vi "Process.vi"(8 "error in":errorcluster, 11 "LockinDAQ":refnum<class "LockinDAQ.lvclass">) -> (0 "error out":errorcluster, 3 "LockinDAQ out":refnum<class "LockinDAQ.lvclass">)   [LabVIEW 2016, in "LockinDAQ.lvclass"]
doc: "---------------------------------------------------------------\nJKI State Machine Objects™\nhttp://jki.net/state-machine-objects/\nCopyright (C) 2005-2015, JKI <info@jki.net>\nALL RIGHTS RESERVED"
uses:
  LockinDAQ.lvclass
  <vilib>/JKI/JKI SMO/SMO/SMO.lvclass
  <vilib>/JKI/JKI SMO/SMO/Typedefs/Parent Call--Enum.ctl
  Typedefs/State-enum.ctl
  Typedefs/Results--Cluster.ctl
  Typedefs/Sample Mode--Ring.ctl
  Typedefs/446xAO-enum.ctl
  Typedefs/DAQType-enum.ctl
  Typedefs/AO.config-cluster.ctl
  Typedefs/AO.config-array.ctl
  Typedefs/PrivateEvents--LockinDAQ.setAOconfig.ctl
  Typedefs/AI.coupling-enum.ctl
  Typedefs/446xAI-enum.ctl
  Typedefs/AI.config-cluster.ctl
  Typedefs/AI.config-array.ctl
  Typedefs/PrivateEvents--LockinDAQ.setAIconfig.ctl
  Typedefs/Function-enum.ctl
  Typedefs/AO-cluster.ctl
  Typedefs/PrivateEvents--LockinDAQ.setAO.ctl
  Typedefs/REF-cluster.ctl
  Typedefs/PrivateEvents--LockinDAQ.setREF.ctl
  Typedefs/Sampling.ctl
  Typedefs/PrivateEvents--LockinDAQ.setSampling.ctl
  Typedefs/Set State-enum.ctl
  Typedefs/PrivateEvents--LockinDAQ.setState.ctl
  Typedefs/PrivateEvents--LockinDAQ.setGain.ctl
  Typedefs/PrivateEvents--Cluster.ctl
  <vilib>/JKI/JKI SMO/SMO/Typedefs/StopProcessEventData--Cluster.ctl
  <vilib>/JKI/JKI SMO/SMO/Typedefs/AbortProcessEventData--Cluster.ctl
  <vilib>/JKI/JKI SMO/SMO/Typedefs/SMO Dependency Event--Enum.ctl
  <vilib>/JKI/JKI SMO/SMO/Typedefs/SMO Dependency Event--Cluster.ctl
  <vilib>/JKI/JKI SMO/SMO/Typedefs/Protected Events.ctl
  <resource>/objmgr/daqmx.rc
  Instrument.Lockin/Instrument.Lockin.lvclass
  Typedefs/PrivateEvents--LockinDAQ.setSweep.ctl
  Typedefs/Sweep Configuration--Cluster.ctl
  Typedefs/SweepResults--Cluster.ctl
  <userlib>/LevyLab/Levylab Instruments/SMOs/LevyLab/LevyLab.lvclass
  Typedefs/PrivateEvents--LockinDAQ.measureOffset.ctl
  Typedefs/PrivateEvents--LockinDAQ.zeroOffset.ctl
  <vilib>/measure/NI_MAPro.lvlib
  Typedefs/PrivateEvents--LockinDAQ.setPreFilter.ctl
  Typedefs/AI Prefilter-cluster.ctl
  C:/Program Files (x86)/National Instruments/LabVIEW 2016/vi.lib/JKI/JKI SMO/SMO/SMO.lvclass
  <vilib>/measure/madcrms.llb/Basic Averaged DC-RMS for N Chan.vi
panel:
  in  "Reset?":bool
  in  "zero offset":bool
  in  "measure offset":bool
  out "State":string
  out "Payload":variant
  out "DAQ Start Tasks (ms)":u32
  out "WFM Generation (ms)":u32
  out "Lockin (ms)":u32
  out "DAQ AO/AI (ms)":u32
  out "DAQ Create Tasks (ms)":u32
  in  "autophase?\n(experimental)":bool
  in  "reset REF":bool
  in  "60 Hz Prefilter?":bool
  in  "LP filter?":bool
  in  "LP Cutoff (Hz)":dbl=0.45 format="%#_13g"
  out "DAQ state":T1=enum."created"
  out "to":i32
  out "Method":string
  # "For instructions on how to use the JKI State Machine Objects, examples and video tutorials, visit:\nhttp://jki.net/state-machine-objects/\n\nJKI State Machine Objects™\nhttp://jki.net/state-machine-objects/\nCopyright (C) 2005-2015, JKI <info@jki.net>\nALL RIGHTS RESERVED"
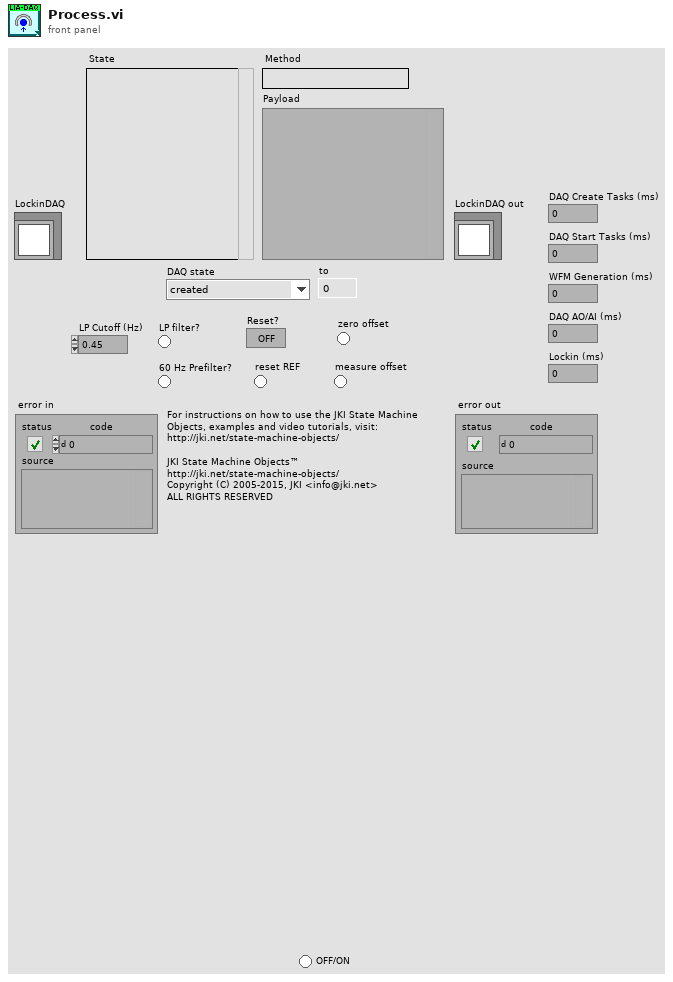
[diagram p1: front panel]
types:
  T1 = typedef "LockinDAQ.lvclass/State-enum.ctl" = enum16{"idle", "created", "started", "stopped", "sweeping"}
  T2 = typedef "SMO.lvclass/Parent Call--Enum.ctl" = enum16{"Allows parent to run", "Does not request parent to run"}
  T3 = enum32{"invalid app kind", "Development System", "Run Time System", "Student Edition", "Embedded LabVIEW", "Evaluation", "Custom"}
  T4 = enum32{"Invalid", "Standard", "Closed", "Hidden", "Minimized", "Maximized"}
  T5 = enum32{"Bad", "Idle", "Run top level", "Running"}
  T6 = typedef "LockinDAQ.lvclass/SweepResults--Cluster.ctl" = cluster{"Time Stamp":timestamp, "X Results":cluster{"parameter":dbl[], "x":dbl[]}[], "Y Results":cluster{"parameter":dbl[], "y":dbl[]}[]}
  T7 = typedef "LockinDAQ.lvclass/Sample Mode--Ring.ctl" = i32
  T8 = typedef "LockinDAQ.lvclass/AO.config-array.ctl" = T9[]
  T9 = typedef "LockinDAQ.lvclass/AO.config-cluster.ctl" = cluster{"AO.channels":tag, "AO.Range":T10, "output terminal configuration":i32, "DAQ Type":T11}
  T10 = typedef "LockinDAQ.lvclass/446xAO-enum.ctl" = enum16{"±0.1 V", "±1.0 V", "±10.0 V"}
  T11 = typedef "LockinDAQ.lvclass/DAQType-enum.ctl" = enum16{"None", "USB 4431", "PXI 446x"}
  T12 = typedef "LockinDAQ.lvclass/Results--Cluster.ctl" = cluster{"Time Stamp":timestamp, "Results":dbl[][]}
  T13 = cluster{"Core":cluster{"Current VI Reference":refnum<vi>, "Close Panel on Exit?":bool, "error":errorcluster}, "Self Reference":refnum<class "LockinDAQ.lvclass">, "to":i32, "state":T1, "sample mode":T7, "AO":waveform(dbl)[], "AI":waveform(dbl)[], "REF":waveform(dbl)[], "Results":T12, "sweep index":i32, "SweepResults [i]":T6, "SweepResults []":T6, "Offset":dbl[]}
  T14 = typedef "LockinDAQ.lvclass/AI.config-array.ctl" = T15[]
  T15 = typedef "LockinDAQ.lvclass/AI.config-cluster.ctl" = cluster{"AI.channels":tag, "AI.Coupling":T16, "AI.Range":T17, "input terminal configuration":i32, "DAQ Type":T11}
  T16 = typedef "LockinDAQ.lvclass/AI.coupling-enum.ctl" = u16
  T17 = typedef "LockinDAQ.lvclass/446xAI-enum.ctl" = enum16{"±0.316 V", "±1.00 V", "±3.16 V", "±10.0 V", "±31.6 V", "±42.4 V"}
  T18 = typedef "LockinDAQ.lvclass/AO-cluster.ctl" = cluster{"Ch":i32[], "Amp (V)":dbl[], "DC (V)":dbl[], "f (Hz)":dbl[], "Phase (°)":dbl[], "Function":T19[], "Sweep?":bool[]}
  T19 = typedef "LockinDAQ.lvclass/Function-enum.ctl" = enum16{"Sine", "Triangle", "Square", "Sawtooth"}
  T20 = typedef "LockinDAQ.lvclass/REF-cluster.ctl" = cluster{"Ch":i32[], " f (Hz)":dbl[], "Phase (°)":dbl[], "TC (s)":dbl[], "order":i32[]}
  T21 = typedef "LockinDAQ.lvclass/PrivateEvents--LockinDAQ.setGain.ctl" = dbl[]
  T22 = typedef "LockinDAQ.lvclass/Sampling.ctl" = cluster{"Fs":dbl, "#s":i32}
  T23 = cluster{"Sampling":T22, "Sample Mode":T7, "AI Buffer Size (S)":i32}
  T24 = typedef "LockinDAQ.lvclass/Sweep Configuration--Cluster.ctl" = cluster{"Sweep Time (s)":dbl, "Initial Wait Time (s)":dbl, "Sweep Channel":i32[], "Sweep Start (V)":dbl[], "Sweep End (V)":dbl[]}
  T25 = typedef "LockinDAQ.lvclass/AI Prefilter-cluster.ctl" = cluster{"60 Hz prefilter":bool, "LP prefilter":bool, "LP cutoff (Hz)":dbl}
  T26 = typedef "LockinDAQ.lvclass/Set State-enum.ctl" = enum16{"start", "stop", "reset", "calibrate", "start sweep", "stop sweep"}
  T27 = cluster{"Current VI Reference":refnum<vi>, "Close Panel on Exit?":bool, "error":errorcluster}
  T28 = typedef "SMO.lvclass/Protected Events.ctl" = cluster{"StopProcesses":refnum<user-event>, "AbortProcesses":refnum<user-event>, "Config Changed":refnum<user-event>, "Dependency":refnum<user-event>}
  T29 = typedef "LockinDAQ.lvclass/PrivateEvents--Cluster.ctl" = cluster{"setAOconfig":refnum<user-event>, "setAIconfig":refnum<user-event>, "setAO":refnum<user-event>, "setREF":refnum<user-event>, "setSampling":refnum<user-event>, "setState":refnum<user-event>, "setGain":refnum<user-event>, "setSweep":refnum<user-event>, "measureOffset":refnum<user-event>, "zeroOffset":refnum<user-event>, "setPreFilter":refnum<user-event>}
  T30 = cluster{"SMO":refnum<event-registration>, "LockinDAQ":refnum<event-registration>, "DAQmx":refnum<event-registration>}
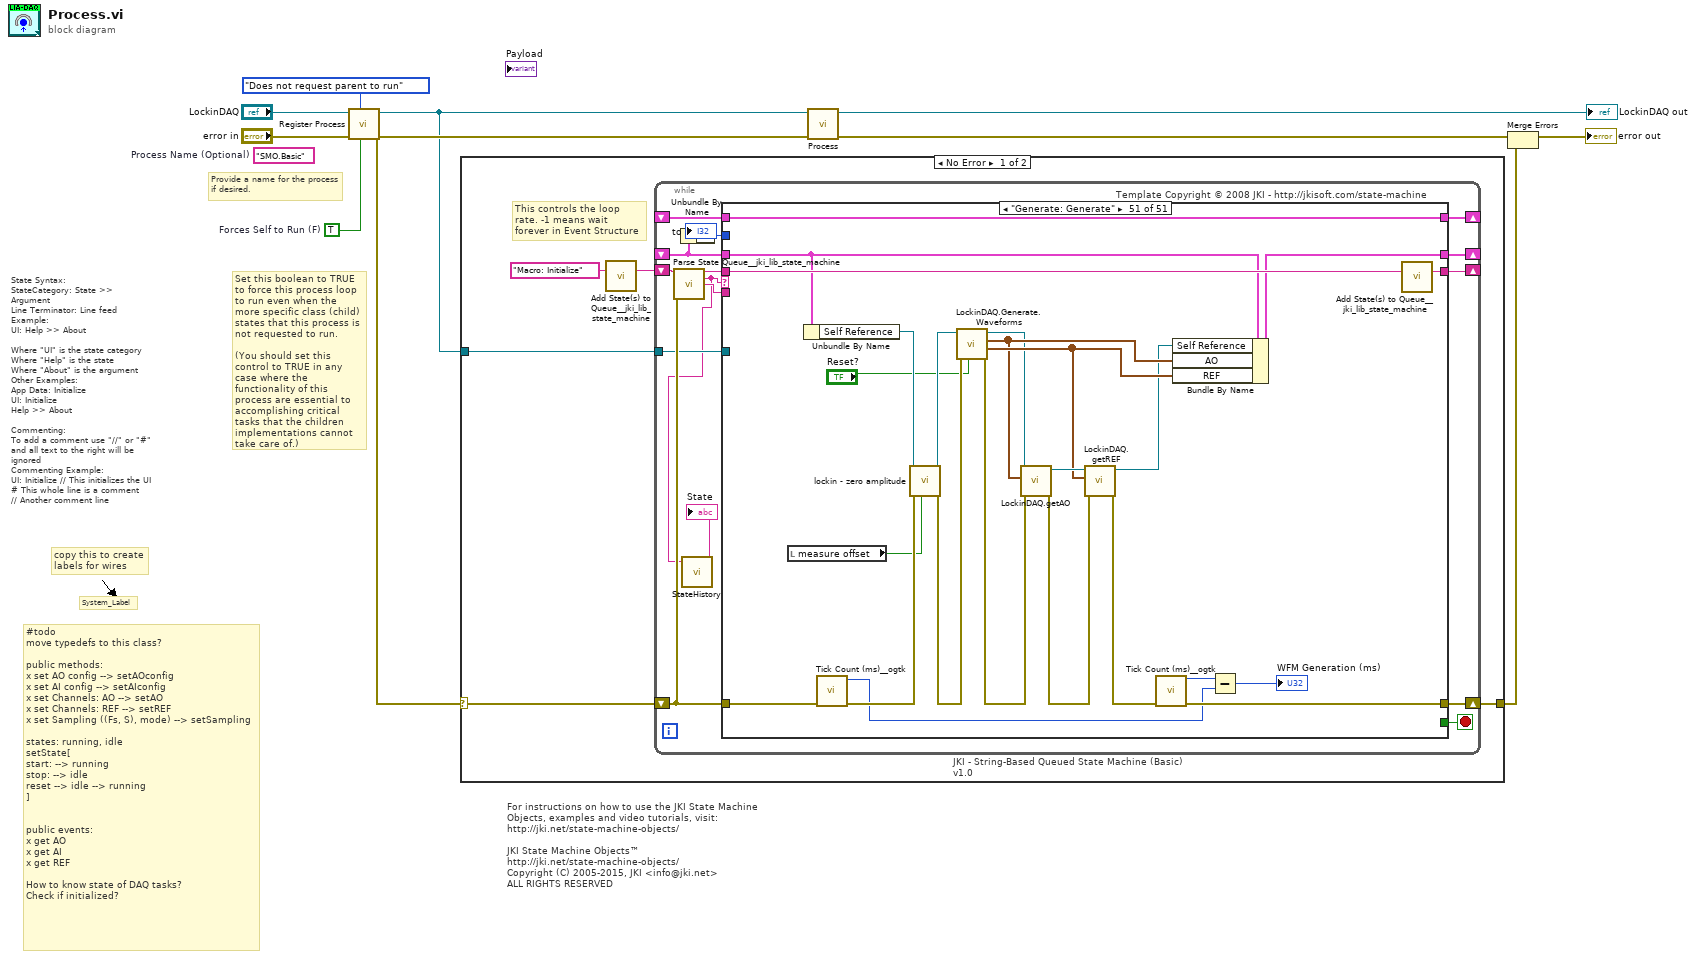
[diagram p0: block diagram]
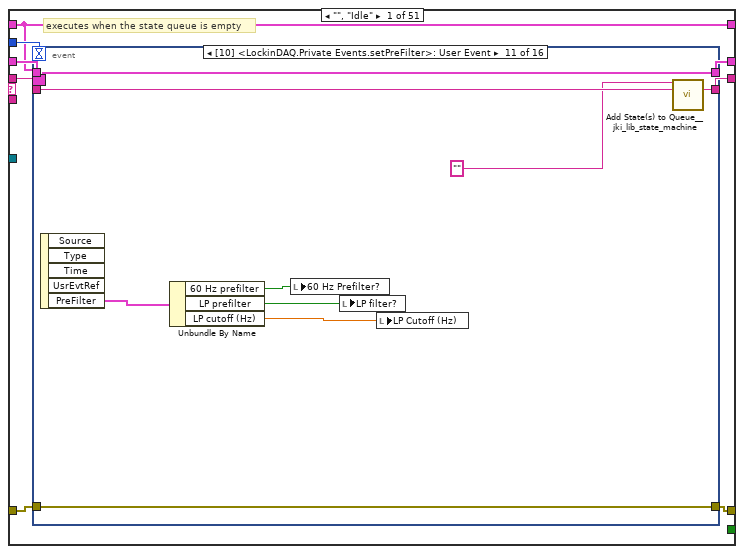
[diagram p2: hidden frame]
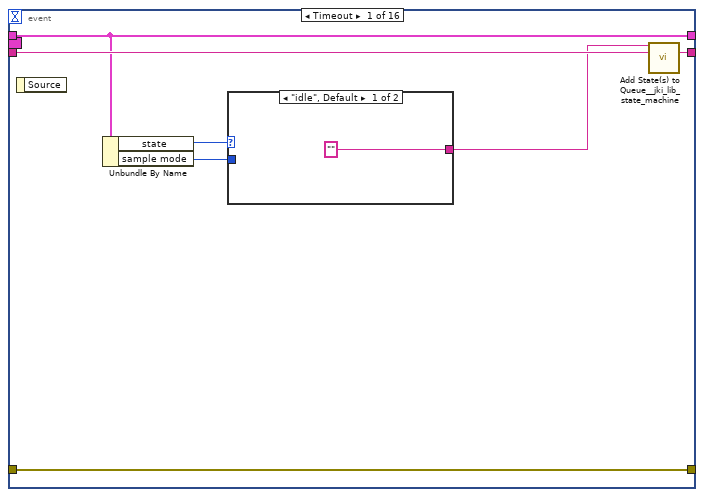
[diagram p3: hidden frame]
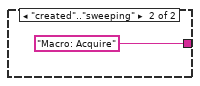
[diagram p4: hidden frame]
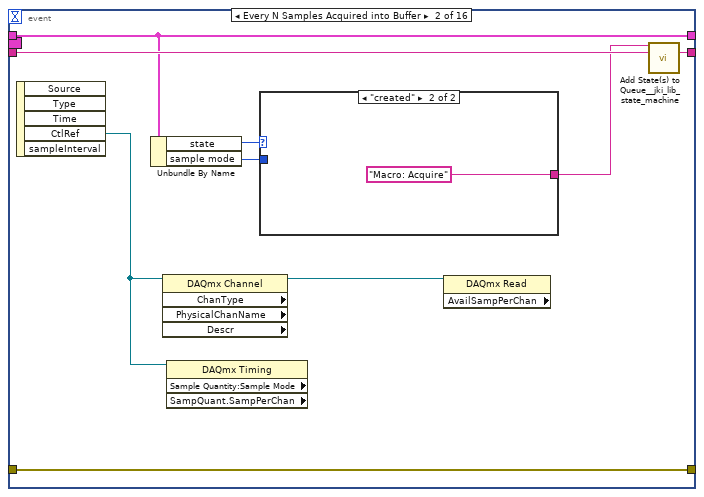
[diagram p5: hidden frame]
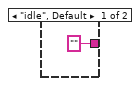
[diagram p6: hidden frame]
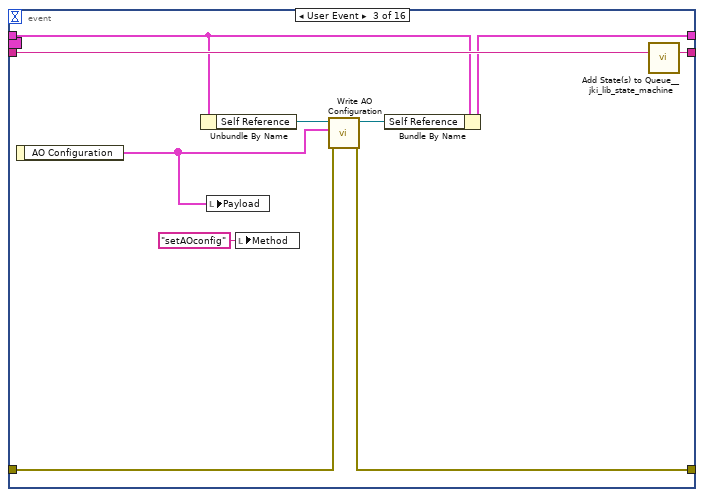
[diagram p7: hidden frame]
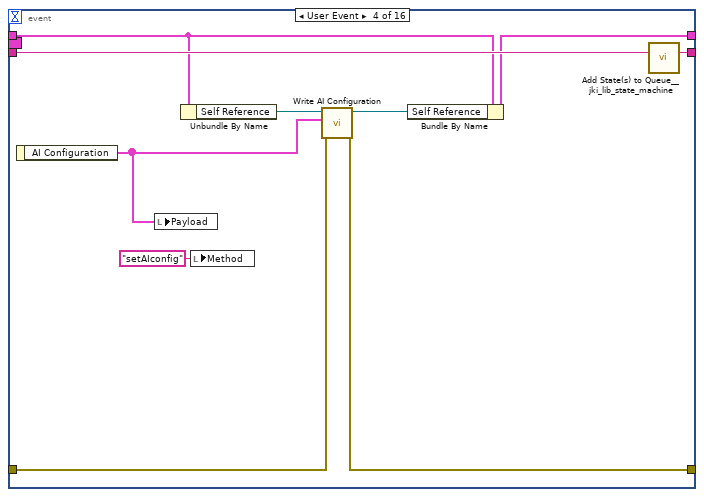
[diagram p8: hidden frame]
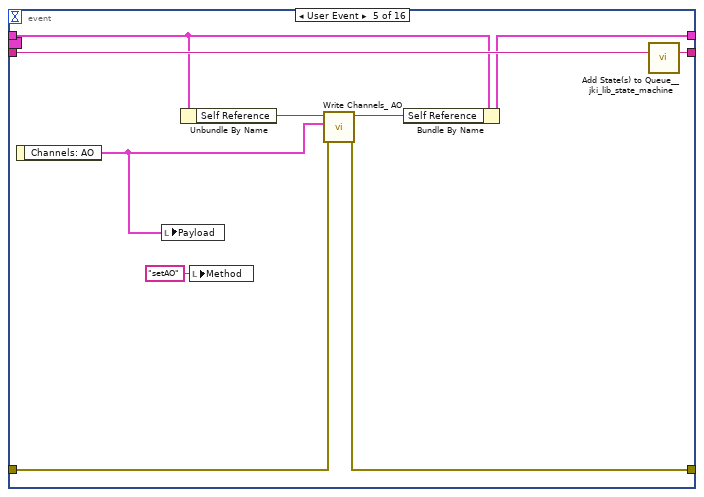
[diagram p9: hidden frame]
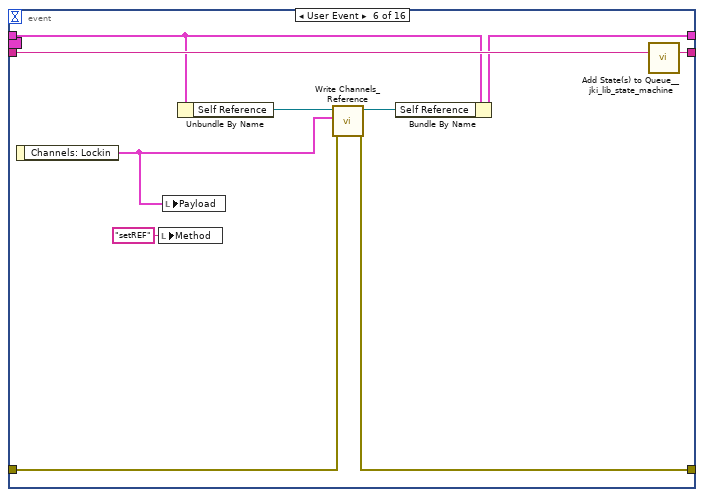
[diagram p10: hidden frame]
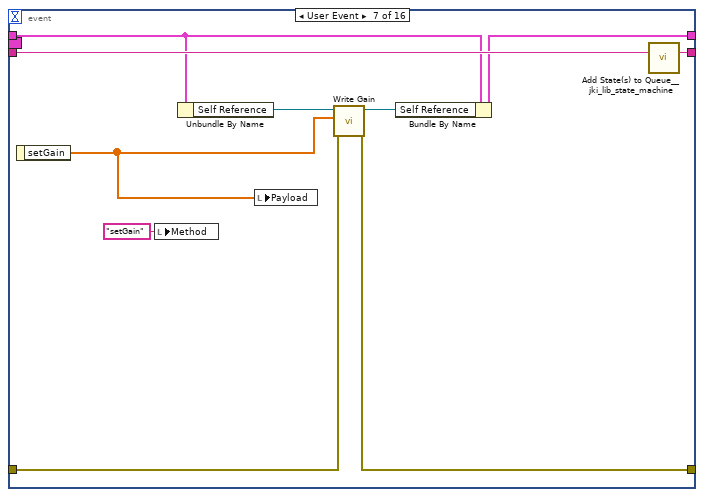
[diagram p11: hidden frame]
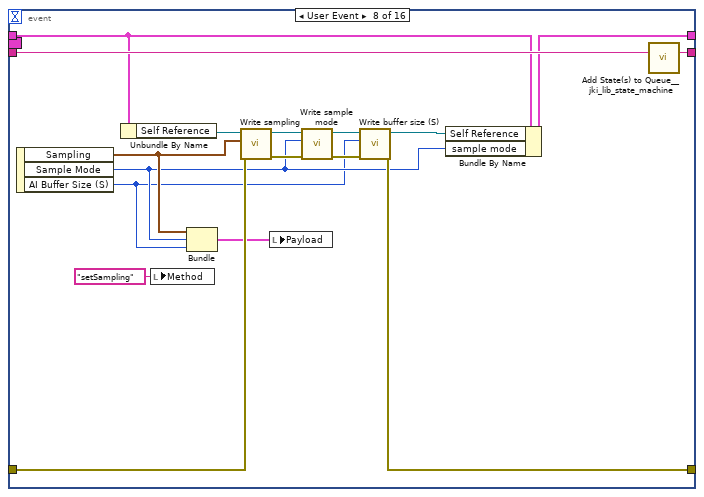
[diagram p12: hidden frame]
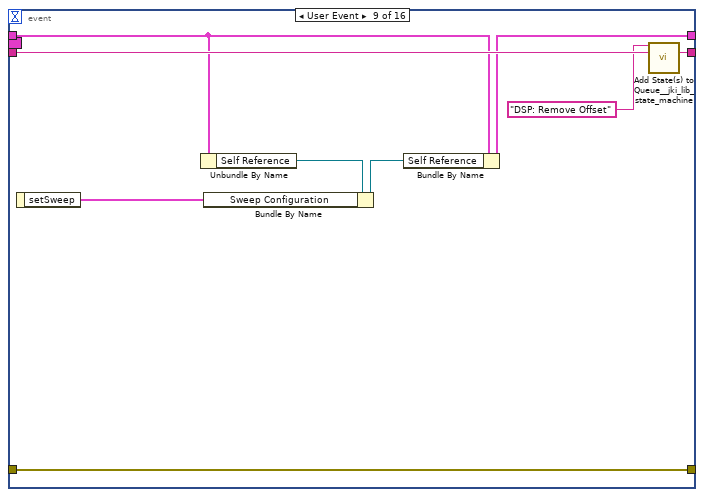
[diagram p13: hidden frame]
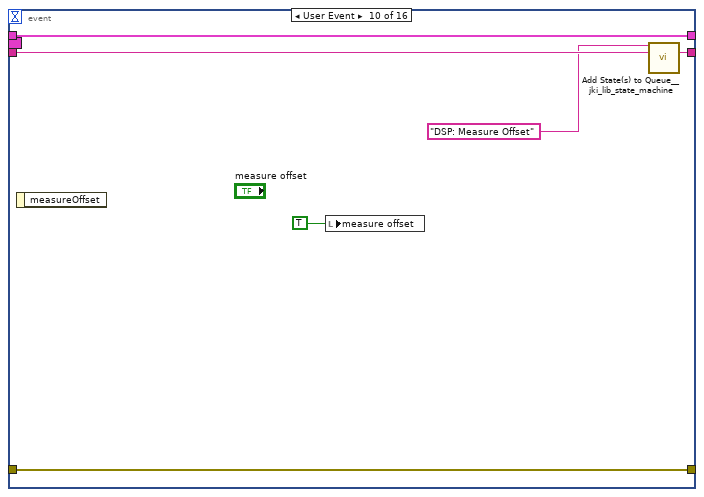
[diagram p14: hidden frame]
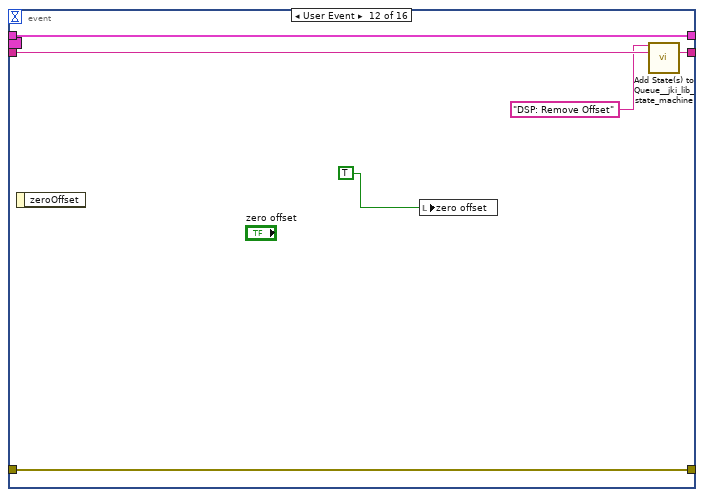
[diagram p15: hidden frame]
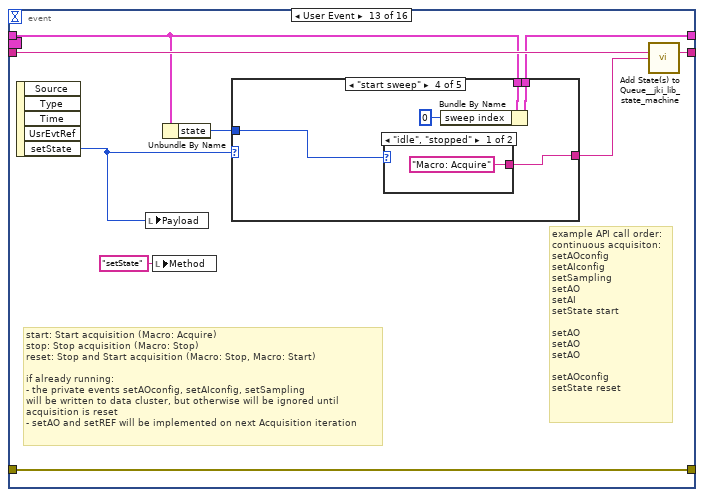
[diagram p16: hidden frame]
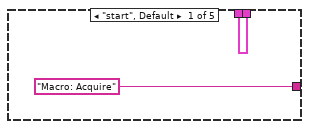
[diagram p17: hidden frame]
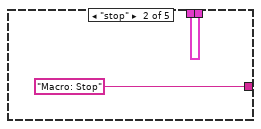
[diagram p18: hidden frame]
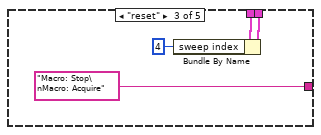
[diagram p19: hidden frame]
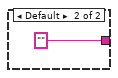
[diagram p20: hidden frame]
diagram:
  w1 = TRUE  # Forces Self to Run (F)
  (unwired) "SMO.Basic"  # Process Name (Optional)
  # "State Syntax:\nStateCategory: State >> Argument\nLine Terminator: Line feed\nExample:\nUI: Help >> About\n\nWhere \"UI\" is the state category\nWhere \"Help\" is the state\nWhere \"About\" is the argument\nOther Examples:\nApp Data: Initialize\nUI: Initialize\nHelp >> About\n\nCommenting:\nTo add a comment use \"//\" or \"#\" and all text to the right will be ignored\nCommenting Example:\nUI: Initialize // This initializes the UI\n# This whole line is a comment\n// Another comment line"
  # "copy this to create labels for wires"
  # "System_Label"
  # "#todo\nmove typedefs to this class?\n\npublic methods:\nx set AO config --> setAOconfig\nx set AI config --> setAIconfig\nx set Channels: AO --> setAO\nx set Channels: REF --> setREF\nx set Sampling ((Fs, S), mode) --> setSampling\n\nstates: running, idle\nsetState[\nstart: --> running\nstop: --> idle\nreset --> idle --> running\n]\n\n\npublic events:\nx get AO\nx get AI\nx get REF\n\nHow to know state of DAQ tasks?\nCheck if initialized?"
  # "Provide a name for the process\nif desired."
  # "Set this boolean to TRUE to force this process loop to run even when the more specific class (child) states that this process is not requested to run.\n\n(You should set this control to TRUE in any case where the functionality of this process are essential to accomplishing critical tasks that the children implementations cannot take care of.)"
  # "For instructions on how to use the JKI State Machine Objects, examples and video tutorials, visit:\nhttp://jki.net/state-machine-objects/\n\nJKI State Machine Objects™\nhttp://jki.net/state-machine-objects/\nCopyright (C) 2005-2015, JKI <info@jki.net>\nALL RIGHTS RESERVED"
  n1 = call <vilib>:"Register Process.vi"("Forces Self to Run (F)"=w1, "Parent Call"=Parent_Call--Enum."Does not request parent to run", "error in (no error)"="error in", "SMO"="LockinDAQ") -> ("error out"=w7:errorcluster, "SMO out"=w6:refnum<class "LockinDAQ.lvclass">)  [unwired: 6 in]
  n2 = case shown="No Error" w7 {
    selector: w7 -> [w14 w939]
    tunnel: w6 -> [w15 _]
    tunnel: [w13 w939] -> w3
    frame No Error {
      # "This controls the loop rate. -1 means wait forever in Event Structure"
      n3 = call <vilib>:"Add State(s) to Queue__jki_lib_state_machine.vi"("State(s) in (\"\")"="Macro: Initialize") -> ("States Out"=w12:string)  [unwired: 14 in]
      n4 = while "JKI - String-Based Queued State Machine (Basic) v1.0" {
        shift-right: [w25] -> _
        shift-left: _ -> [w19]
        shift-right: [w18] -> w13
        shift-left: w14 -> [w24]
        shift-right: [w27] -> _
        shift-left: w12 -> [w28]
        tunnel: w15 -> [w23]
        shift-right: [w22] -> _
        shift-left: _ -> [w21]
        stop <- w26 stop-if-true
        # "Template Copyright © 2008 JKI - http://jkisoft.com/state-machine"
        n5 = call <vilib>:"Parse State Queue__jki_lib_state_machine.vi"("State Queue"=w28, "Error In (no error)"=w24) -> ("Remaining States"=w30:string, "Current State"=w17:string, "Arguments"=w29:string)  [unwired: 11 in]
        n6 = Unbundle By Name(w19) -> ("to"=w20:i32)
        "to" <- w20
        n7 = call "StateHistory.vi"("Current State in"=w17) -> ("State History"=→"State":string)  [unwired: 8 in, 1 out]
        n8 = case shown="\"Generate: Generate\"" w17 {
          selector: w17 -> [_ _ w206 _ _ _ _ _ _ _ _ _ _ _ _ _ _ _ _ _ _ _ _ _ _ _ _ _ _ _ _ _ _ _ _ _ _ _ _ _ _ _ _ _ _ _ _ _ _ _ _]
          tunnel: w30 -> [w38 w204 w210 w229 w233 w254 w259 w281 w288 w293 w299 w306 w322 w354 w368 w382 w395 w405 w413 w421 w433 w438 w449 w454 w477 w483 w488 w505 w545 w583 w592 w602 w623 w660 w672 w677 w695 w738 w774 w789 w798 w804 w819 w828 w842 w854 w873 w892 w909 w914 w938]
          tunnel: w29 -> [_ _ _ _ _ _ _ _ _ _ _ w300 w316 _ _ _ _ _ _ _ _ _ _ _ _ _ _ _ _ _ _ w597 _ _ _ _ _ _ _ _ _ _ _ _ _ _ _ _ _ _ _]
          tunnel: w19 -> [w36 w201 w208 w220 w246 w250 w256 _ w283 w290 w297 w304 w318 w351 w364 w374 w390 w402 w406 w418 w431 w435 w446 w451 w475 w481 w486 w502 w542 w580 w590 w599 w620 w657 w663 w675 w682 w735 w771 w786 w792 w802 w816 w825 w831 w851 w859 w888 w905 w912 w934]
          tunnel: w24 -> [w34 w202 w211 w226 w239 _ w257 w279 w285 w291 w296 w302 w320 w352 w366 w380 w393 w403 w411 w414 w432 w436 w441 w452 w473 w480 w484 w499 w539 w578 w585 w594 w617 w654 w665 w673 w680 w723 w769 w777 w795 w800 w810 w823 w839 w848 w870 w883 w898 w910 w925]
          tunnel: [w37 w203 w209 w228 w230 w253 w258 w280 w287 w292 w298 w305 w321 w353 w367 w381 w394 w404 w412 w420 w429 w437 w448 w453 w476 w482 w487 w504 w544 w582 w591 w601 w622 w659 w671 w676 w694 w737 w773 w788 w797 w803 w818 w827 w841 w853 w872 w891 w908 w913 w937] -> w27
          tunnel: [_ _ _ _ _ TRUE _ _ _ _ _ _ _ _ _ _ _ _ _ _ _ _ _ _ _ _ _ _ _ _ _ _ _ _ _ _ _ _ _ _ _ _ _ _ _ _ _ _ _ _ _] -> w26
          tunnel: [w33 w201 w208 w227 w245 w250 w256 w270 w283 w290 w297 w304 w318 w351 w364 w374 w390 w402 w406 w418 w431 w435 w446 w451 w475 w481 w486 w501 w541 w579 w589 w598 w619 w656 w662 w675 w681 w734 w770 w785 w794 w802 w815 w824 w830 w850 w858 w889 w906 w912 w933] -> w25
          tunnel: w20 -> [w32 _ _ _ _ _ _ _ _ _ _ _ _ _ _ _ _ _ _ _ _ _ _ _ _ _ _ _ _ _ _ _ _ _ _ _ _ _ _ _ _ _ _ _ _ _ _ _ _ _ _]
          tunnel: w23 -> [_ _ _ _ _ _ _ w277 _ _ _ _ _ _ _ _ _ _ _ _ _ _ _ _ _ _ _ _ _ _ _ _ _ _ _ _ _ _ _ _ _ _ _ _ _ _ _ _ _ _ _]
          tunnel: [w31 w200 w205 w217 w248 w251 w255 w276 w282 w289 w295 w303 w315 w350 w365 w375 w392 w401 w410 w419 w430 w434 w447 w450 w468 w478 w485 w503 w543 w581 w588 w600 w621 w658 w669 w674 w693 w736 w772 w787 w796 w801 w817 w826 w840 w852 w871 w890 w907 w911 w936] -> w22
          tunnel: w21 -> [w31 w200 w205 w217 w248 w251 w255 w276 w282 w289 w295 w303 w315 w350 w365 w375 w392 w401 w410 w419 w430 w434 w447 w450 _ w478 w485 w503 w543 w581 w588 w600 w621 w658 w668 w674 w693 w736 w772 w787 w796 w801 w817 w826 w840 w852 w871 w890 w907 w911 w936]
          tunnel: [w35 w202 w212 w226 w247 w249 w257 w265 w284 w291 w296 w301 w319 w352 w366 w380 w393 w403 w411 w414 w432 w436 w440 w452 w472 w480 w484 w498 w538 w572 w584 w593 w612 w648 w664 w673 w679 w727 w763 w782 w795 w800 w814 w820 w839 w846 w870 w882 w904 w910 w920] -> w18
          frame "", "Idle" {
            # "executes when the state queue is empty"
            n9 = event shown="[10] <LockinDAQ.Private Events.setPreFilter>: User Event" {
              selector: w31 -> [_ _ _ _ _ _ _ _ _ _ _ _ _ _ _ _]
              dyn-events: _ -> [_ _ _ _ _ _ _ _ _ _ _ _ _ _ _ _]
              timeout: w32 -> [_ _ _ _ _ _ _ _ _ _ _ _ _ _ _ _]
              tunnel: w38 -> [w45 w56 w68 w78 w88 w98 w108 w125 w134 w140 w149 w155 w164 w189 w194 w199]
              tunnel: [w44 w55 w67 w77 w87 w97 w107 w124 w133 w139 w148 w154 w163 w188 w193 w198] -> w37
              tunnel: w36 -> [w42 w53 w64 w74 w84 w94 w104 w121 w130 w136 w145 w152 w157 w186 w191 w196]
              tunnel: [w43 w54 w60 w70 w80 w90 w101 w113 w131 w138 w147 w153 w162 w187 w192 w197] -> w35
              tunnel: w34 -> [w43 w54 w61 w71 w81 w91 w102 w117 w131 w138 w147 w153 w162 w187 w192 w197]
              tunnel: [w42 w53 w66 w76 w86 w96 w106 w123 w132 w136 w145 w152 w156 w186 w191 w196] -> w33
              event Timeout {
                n10 = event-data() -> ()  [unwired: 1 in, 1 out]
                n11 = Unbundle By Name(w42) -> ("state"=w40:T1, "sample mode"=w41:T7)
                n12 = case shown="\"idle\", Default" w40 {
                  tunnel: w41 -> [_ _]
                  tunnel: ["" ("State(s) in Front (\"\")") "Macro: Acquire" ("State(s) in Front (\"\")")] -> w39
                  frame "idle", Default {
                  }
                  frame "created".."sweeping" {
                  }
                }
                n13 = call <vilib>:"Add State(s) to Queue__jki_lib_state_machine.vi"("State(s) in Front (\"\")"=w39, "State(s) in (\"\")"=w45) -> ("States Out"=w44:string)  [unwired: 13 in]
              }
              event Every N Samples Acquired into Buffer {
                n14 = event-data() -> ("CtlRef"=w49:refnum<k21>)  [unwired: 1 in, 4 out]
                n15 = Unbundle By Name(w53) -> ("state"=w50:T1, "sample mode"=w52:T7)
                n16 = property class="DAQmx Channel" props=["ChanType", "PhysicalChanName", "Descr"](reference=w49) -> (reference out=w48:refnum<k21>)  [unwired: 1 in, 4 out]
                n17 = property class="DAQmx Timing" props=["Sample Quantity:Sample Mode", "SampQuant.SampPerChan"](reference=w49) -> ()  [unwired: 1 in, 4 out]
                n18 = case shown="\"created\"" w50 {
                  tunnel: w52 -> [_ _]
                  tunnel: ["" ("State(s) in Front (\"\")") "Macro: Acquire" ("State(s) in Front (\"\")")] -> w51
                  frame "idle", Default {
                  }
                  frame "created" {
                  }
                }
                n19 = property class="DAQmx Read" props=["AvailSampPerChan"](reference=w48) -> ()  [unwired: 1 in, 3 out]
                n20 = call <vilib>:"Add State(s) to Queue__jki_lib_state_machine.vi"("State(s) in Front (\"\")"=w51, "State(s) in (\"\")"=w56) -> ("States Out"=w55:string)  [unwired: 13 in]
              }
              event User Event {
                n21 = event-data() -> ("AO Configuration"=w59:T8)  [unwired: 1 in]
                n22 = Unbundle By Name(w64) -> ("Self Reference"=w63:refnum<class "LockinDAQ.lvclass">)
                n23 = local write "Payload"(w59) -> ()
                n24 = local write "Method"("setAOconfig" ("String")) -> ()
                n25 = call "Write AO Configuration.vi"("error in (no error)"=w61, "AO Configuration"=w59, "LockinDAQ"=w63) -> ("error out"=w60:errorcluster, "LockinDAQ out"=w62:refnum<class "LockinDAQ.lvclass">)  [unwired: 7 in]
                n26 = Bundle By Name(cluster=w64, "Self Reference"=w62) -> (w66:T13)
                n27 = call <vilib>:"Add State(s) to Queue__jki_lib_state_machine.vi"("State(s) in (\"\")"=w68) -> ("States Out"=w67:string)  [unwired: 14 in]
              }
              event User Event {
                n28 = event-data() -> ("AI Configuration"=w69:T14)  [unwired: 1 in]
                n29 = local write "Payload"(w69) -> ()
                n30 = Unbundle By Name(w74) -> ("Self Reference"=w73:refnum<class "LockinDAQ.lvclass">)
                n31 = local write "Method"("setAIconfig" ("String")) -> ()
                n32 = call "Write AI Configuration.vi"("error in (no error)"=w71, "AI Configuration"=w69, "LockinDAQ"=w73) -> ("error out"=w70:errorcluster, "LockinDAQ out"=w72:refnum<class "LockinDAQ.lvclass">)  [unwired: 7 in]
                n33 = Bundle By Name(cluster=w74, "Self Reference"=w72) -> (w76:T13)
                n34 = call <vilib>:"Add State(s) to Queue__jki_lib_state_machine.vi"("State(s) in (\"\")"=w78) -> ("States Out"=w77:string)  [unwired: 14 in]
              }
              event User Event {
                n35 = event-data() -> ("Channels: AO"=w79:T18)  [unwired: 1 in]
                n36 = local write "Payload"(w79) -> ()
                n37 = Unbundle By Name(w84) -> ("Self Reference"=w82:refnum<class "LockinDAQ.lvclass">)
                n38 = local write "Method"("setAO" ("String")) -> ()
                n39 = call "Write Channels_ AO.vi"("error in (no error)"=w81, "Channels: AO"=w79, "LockinDAQ"=w82) -> ("error out"=w80:errorcluster, "LockinDAQ out"=w83:refnum<class "LockinDAQ.lvclass">)  [unwired: 7 in]
                n40 = Bundle By Name(cluster=w84, "Self Reference"=w83) -> (w86:T13)
                n41 = call <vilib>:"Add State(s) to Queue__jki_lib_state_machine.vi"("State(s) in (\"\")"=w88) -> ("States Out"=w87:string)  [unwired: 14 in]
              }
              event User Event {
                n42 = event-data() -> ("Channels: Lockin"=w89:T20)  [unwired: 1 in]
                n43 = local write "Method"("setREF" ("String")) -> ()
                n44 = local write "Payload"(w89) -> ()
                n45 = Unbundle By Name(w94) -> ("Self Reference"=w93:refnum<class "LockinDAQ.lvclass">)
                n46 = call "Write Channels_ Reference.vi"("error in (no error)"=w91, "Channels: Lockin"=w89, "LockinDAQ"=w93) -> ("error out"=w90:errorcluster, "LockinDAQ out"=w92:refnum<class "LockinDAQ.lvclass">)  [unwired: 7 in]
                n47 = Bundle By Name(cluster=w94, "Self Reference"=w92) -> (w96:T13)
                n48 = call <vilib>:"Add State(s) to Queue__jki_lib_state_machine.vi"("State(s) in (\"\")"=w98) -> ("States Out"=w97:string)  [unwired: 14 in]
              }
              event User Event {
                n49 = event-data() -> ("setGain"=w99:T21)  [unwired: 1 in]
                n50 = local write "Method"("setGain" ("String")) -> ()
                n51 = Unbundle By Name(w104) -> ("Self Reference"=w103:refnum<class "LockinDAQ.lvclass">)
                n52 = local write "Payload"(w99) -> ()
                n53 = call "Write Gain.vi"("error in (no error)"=w102, "Gain"=w99, "LockinDAQ"=w103) -> ("error out"=w101:errorcluster, "LockinDAQ out"=w100:refnum<class "LockinDAQ.lvclass">)  [unwired: 7 in]
                n54 = Bundle By Name(cluster=w104, "Self Reference"=w100) -> (w106:T13)
                n55 = call <vilib>:"Add State(s) to Queue__jki_lib_state_machine.vi"("State(s) in (\"\")"=w108) -> ("States Out"=w107:string)  [unwired: 14 in]
              }
              event User Event {
                n56 = event-data() -> ("Sampling"=w112:T22, "Sample Mode"=w111:T7, "AI Buffer Size (S)"=w110:i32)  [unwired: 1 in]
                n57 = Unbundle By Name(w121) -> ("Self Reference"=w120:refnum<class "LockinDAQ.lvclass">)
                n58 = local write "Method"("setSampling" ("String")) -> ()
                n59 = Bundle("Sampling"=w112, "Sample Mode"=w111, "AI Buffer Size (S)"=w110) -> (w109:T23)  [unwired: 1 in]
                n60 = call "Write sampling.vi"("error in (no error)"=w117, "sampling"=w112, "LockinDAQ"=w120) -> ("error out"=w118:errorcluster, "LockinDAQ out"=w119:refnum<class "LockinDAQ.lvclass">)  [unwired: 7 in]
                n61 = local write "Payload"(w109) -> ()
                n62 = call "Write sample mode.vi"("error in (no error)"=w118, "sample mode"=w111, "LockinDAQ"=w119) -> ("error out"=w114:errorcluster, "LockinDAQ out"=w116:refnum<class "LockinDAQ.lvclass">)  [unwired: 7 in]
                n63 = call "Write buffer size (S).vi"("error in (no error)"=w114, "buffer size (S)"=w110, "LockinDAQ"=w116) -> ("error out"=w113:errorcluster, "LockinDAQ out"=w115:refnum<class "LockinDAQ.lvclass">)  [unwired: 7 in]
                n64 = Bundle By Name(cluster=w121, "Self Reference"=w115, "sample mode"=w111) -> (w123:T13)
                n65 = call <vilib>:"Add State(s) to Queue__jki_lib_state_machine.vi"("State(s) in (\"\")"=w125) -> ("States Out"=w124:string)  [unwired: 14 in]
              }
              event User Event {
                n66 = event-data() -> ("setSweep"=w127:T24)  [unwired: 1 in]
                n67 = Unbundle By Name(w130) -> ("Self Reference"=w129:refnum<class "LockinDAQ.lvclass">)
                n68 = Bundle By Name(cluster=w129, "Sweep Configuration"=w127) -> (w128:refnum<class "LockinDAQ.lvclass">)
                n69 = Bundle By Name(cluster=w130, "Self Reference"=w128) -> (w132:T13)
                n70 = call <vilib>:"Add State(s) to Queue__jki_lib_state_machine.vi"("State(s) in Front (\"\")"="DSP: Remove Offset" ("State(s) in Front (\"\")"), "State(s) in (\"\")"=w134) -> ("States Out"=w133:string)  [unwired: 13 in]
              }
              event User Event {
                n71 = event-data() -> ()  [unwired: 1 in, 1 out]
                n72 = local write "measure offset"(TRUE ("measureOffset")) -> ()
                n73 = call <vilib>:"Add State(s) to Queue__jki_lib_state_machine.vi"("State(s) in Front (\"\")"="DSP: Measure Offset" ("State(s) in Front (\"\")"), "State(s) in (\"\")"=w140) -> ("States Out"=w139:string)  [unwired: 13 in]
              }
              event User Event {
                n74 = event-data() -> ("PreFilter"=w144:T25)  [unwired: 1 in, 4 out]
                n75 = Unbundle By Name(w144) -> ("60 Hz prefilter"=w143:bool, "LP prefilter"=w142:bool, "LP cutoff (Hz)"=w141:dbl)
                n76 = local write "60 Hz Prefilter?"(w143) -> ()
                n77 = local write "LP filter?"(w142) -> ()
                n78 = local write "LP Cutoff (Hz)"(w141) -> ()
                n79 = call <vilib>:"Add State(s) to Queue__jki_lib_state_machine.vi"("State(s) in Front (\"\")"="" ("State(s) in Front (\"\")"), "State(s) in (\"\")"=w149) -> ("States Out"=w148:string)  [unwired: 13 in]
              }
              event User Event {
                n80 = event-data() -> ()  [unwired: 1 in, 1 out]
                n81 = local write "zero offset"(TRUE ("zero offset")) -> ()
                n82 = call <vilib>:"Add State(s) to Queue__jki_lib_state_machine.vi"("State(s) in Front (\"\")"="DSP: Remove Offset" ("State(s) in Front (\"\")"), "State(s) in (\"\")"=w155) -> ("States Out"=w154:string)  [unwired: 13 in]
              }
              event User Event {
                # "example API call order:\ncontinuous acquisiton:\nsetAOconfig\nsetAIconfig\nsetSampling\nsetAO\nsetAI\nsetState start\n\nsetAO\nsetAO\nsetAO\n\nsetAOconfig\nsetState reset"
                # "start: Start acquisition (Macro: Acquire)\nstop: Stop acquisition (Macro: Stop)\nreset: Stop and Start acquisition (Macro: Stop, Macro: Start)\n\nif already running:\n- the private events setAOconfig, setAIconfig, setSampling\nwill be written to data cluster, but otherwise will be ignored until\nacquisition is reset\n- setAO and setREF will be implemented on next Acquisition iteration"
                n83 = event-data() -> ("setState"=w158:T26)  [unwired: 1 in, 4 out]
                n84 = local write "Payload"(w158) -> ()
                n85 = local write "Method"("setState" ("String")) -> ()
                n86 = Unbundle By Name(w157) -> ("state"=w159:T1)
                n87 = case shown="\"start sweep\"" w158 {
                  tunnel: ["Macro: Acquire" ("State(s) in Front (\"\")") "Macro: Stop" ("State(s) in Front (\"\")") "Macro: Stop\nMacro: Acquire" ("State(s) in Front (\"\")") w175 "" ("State(s) in Front (\"\")")] -> w160
                  tunnel: w159 -> [_ _ _ w173 _]
                  tunnel: w157 -> [w165 w167 w172 w177 w183]
                  tunnel: [w165 w167 w171 w176 w182] -> w156
                  frame "start", Default {
                  }
                  frame "stop" {
                  }
                  frame "reset" {
                    n88 = Bundle By Name(cluster=w172, "sweep index"=4) -> (w171:T13)
                  }
                  frame "start sweep" {
                    n89 = case shown="\"idle\", \"stopped\"" w173 {
                      tunnel: ["Macro: Acquire" ("State(s) in Front (\"\")") "" ("State(s) in Front (\"\")")] -> w175
                      frame "idle", "stopped" {
                      }
                      frame Default {
                      }
                    }
                    n90 = Bundle By Name(cluster=w177, "sweep index"=0) -> (w176:T13)
                  }
                  frame "stop sweep" {
                    n91 = Bundle By Name(cluster=w183, "sweep index"=4) -> (w182:T13)
                  }
                }
                n92 = call <vilib>:"Add State(s) to Queue__jki_lib_state_machine.vi"("State(s) in (\"\")"=w164, "State(s) at Back (\"\")"=w160) -> ("States Out"=w163:string)  [unwired: 13 in]
              }
              event Panel Close? {
                # "Discard the event because we'll close the front panel ourselves in Macro: Exit"
                # "Close Panel button (pressed) Event\n(this executes Macro: Exit to terminate the VI)"
                n93 = event-data() -> ()  [unwired: 1 in, 1 out]
                n94 = event-data("Discard?"=FALSE) -> ()  [unwired: 1 in, 1 out]
                n95 = call <vilib>:"Add State(s) to Queue__jki_lib_state_machine.vi"("State(s) in Front (\"\")"="//Macro: Exit", "State(s) in (\"\")"=w189) -> ("States Out"=w188:string)  [unwired: 13 in]
              }
              event User Event {
                n96 = event-data() -> ()  [unwired: 1 in, 5 out]
                n97 = call <vilib>:"Add State(s) to Queue__jki_lib_state_machine.vi"("State(s) in Front (\"\")"="Macro: Exit", "State(s) in (\"\")"=w194) -> ("States Out"=w193:string)  [unwired: 13 in]
              }
              event User Event {
                # "On Abort, no nice macro exit, but exit right away"
                n98 = event-data() -> ()  [unwired: 1 in, 5 out]
                n99 = call <vilib>:"Add State(s) to Queue__jki_lib_state_machine.vi"("State(s) in Front (\"\")"="Exit", "State(s) in (\"\")"=w199) -> ("States Out"=w198:string)  [unwired: 13 in]
              }
            }
          }
          frame "---------- Core ----------" {
            # "Do not put any code in this frame.\n(it is a separator no-op)"
            n100 = call <vilib>:"Add State(s) to Queue__jki_lib_state_machine.vi"("State(s) in (\"\")"=w204) -> ("States Out"=w203:string)  [unwired: 14 in]
          }
          frame Default {
            w215 = 42 items=["No error", "Argument error", "Memory is full", "Out of zone", "End of file", "File already open", "Generic file I/O error", "File not found", "File permission error", "Disk is full", "Duplicate path", "Too many files open", "System feature not enabled", "Resource file not found", "Cannot add resource", "Resource not found", "Image not found", "Image memory error", "Pen does not exist", "Config type invalid", "Config token not found", "Config parse error", "Config memory error", "Bad external code format", "Bad external code offset", "External code not present", "Null window", "Destroy window error", "Null menu", "Print aborted", "Bad print record", "Print driver error", "Windows error during printing", "Memory error during printing", "Print dialog error", "Generic print error", "Invalid device refnum", "Device not found", "Device parameter error", "Device unit error", "Cannot open device", "Device call aborted", "Generic error", "Cancelled by user", "Object ID too low", "Object ID too high", "Object not in heap", "Unknown heap", "Unknown object (invalid DefProc)", "Unknown object (DefProc not in table)", "Message out of range", "Invalid (null) method", "Unknown message", "Manager call not supported", "Bad address", "Network operation in progress", "Network operation timed out", "Connection is busy", "Network attribute not supported", "Network error", "Address in use", "System out of memory", "Connection aborted", "Connection refused", "Not connected", "Already connected", "Connection closed", "Initialization error (interapplication manager)", "Bad occurrence", "Wait on unbound occurrence handler", "Occurrence queue overflow", "Datalog type conflict", "Unused", "Unrecognized type (interapplication manager)", "Memory corrupt", "Failed to make temporary DLL", "Old CIN version", "Drag socket not found", "Failed to load drop-object", "Failed to register OLE object", "Failed to release OLE object", "Format specifier type mismatch", "Unknown format specifier", "Too few format specifiers", "Too many format specifiers", "Scan failed", "Newer CIN version", "Error converting to variant", "Runtime menu error", "Password tampered", "Variant attribute not found", "Incompatible variant data type", "Event data is not available", "Event Store is not present", "Occurrence is not found", "Event Queue is not created", "Event info is not available", "Refnum passed is NULL", "Error retrieving Class GUID", "Error retrieving CoClass GUID", "Error retrieving TypeLib GUID.", "Bad built application magic bytes.", "Specific driver is different from the specific driver associated with the Logical Name.", "There is no session opened to the class driver.", "Max Error", "MAX - Error with config objects", "MAX - Error loading configuration", "MAX - Group not supported"]
            # "Current State"
            # "Do not delete, rename, or modify this frame.\n(this is used to capture unhandled states and typos)"
            # "Handle mistyped state name (developer tool)"
            n101 = Format Into String(format string="Software Exception: Unhandled State \"%s\"." ("message"), error in=w211, w206) -> (resulting string=w214:string, error out=w213:errorcluster)  [unwired: 1 in]
            n102 = call <vilib>:"Error Cluster From Error Code.vi"("show call chain? (False)"=TRUE, "error in (no error)"=w213, "error message (\"\")"=w214, "error code (0)"=w215) -> ("error out"=w212:errorcluster)  [unwired: 5 in]
            n103 = call <vilib>:"Add State(s) to Queue__jki_lib_state_machine.vi"("State(s) in (\"\")"=w210) -> ("States Out"=w209:string)  [unwired: 14 in]
          }
          frame "Initialize Core Data" {
            # "Do not delete, rename, or modify this frame.\n(this is used to determine panel behavior on exit)"
            # "originally closed?"
            # "exe?"
            # "If panel starts closed or is an EXE, then close it when we exit"
            n104 = property class="App"() -> ("App.Kind"=w224:T3)  [unwired: 2 in, 2 out]
            n105 = property class="VI"() -> ("Front Panel.Open"=w225:bool)  [unwired: 2 in, 2 out]
            n106 = control-ref of="Current VI Reference"() -> (w218:refnum<vi>)
            n107 = Not(x=w225) -> (.not. x?=w222:bool)
            n108 = Equal?(x=w224, y=T3."Run Time System" ("Application:Kind")) -> (x = y?=w221:bool)
            n109 = Or(x=w222, y=w221) -> (x .or. y?=w219:bool)
            n110 = Bundle By Name(cluster=w220, "Core.Current VI Reference"=w218, "Core.Close Panel on Exit?"=w219) -> (w227:T13)
            n111 = call <vilib>:"Add State(s) to Queue__jki_lib_state_machine.vi"("State(s) in (\"\")"=w229) -> ("States Out"=w228:string)  [unwired: 14 in]
          }
          frame "Error Handler" {
            w240 = FALSE  # Stop on Unhandled Error (T)
            w247 = errorcluster {"status"=FALSE, "code"=0, "source"=""}  # No error
            # "Overwrite this method to handle errors and pass to parent if not handled. Parent will fire a public event if the error is not handled up the chain of classes."
            n112 = Unbundle By Name(w246) -> ("Self Reference"=w237:refnum<class "LockinDAQ.lvclass">)
            n113 = call "LockinDAQ.ErrorHandler.vi"("error in (no error)"=w239, "LockinDAQ in"=w237) -> ("error out"=w238:errorcluster, "Error Filtered?"=w235:bool, "LockinDAQ out"=w236:refnum<class "LockinDAQ.lvclass">)  [unwired: 6 in, 1 out]
            n114 = call-dynamic "Handle Error.vi"("Stop on Unhandled Error (T)"=w240, "error in"=w238, "LevyLab"=w236) -> ("handling error"=w241:errorcluster, "Unhandled error"=w244:errorcluster)  [unwired: 6 in, 1 out]
            n115 = Bundle By Name(cluster=w246, "Core.error"=w244) -> (w245:T13)
            n116 = Select(t="Exit", s=w241, f="") -> (s? t:f=w232:string)
            n117 = call <vilib>:"Add State(s) to Queue__jki_lib_state_machine.vi"("State(s) in Front (\"\")"=w232, "State(s) in (\"\")"=w233) -> ("States Out"=w231:string)  [unwired: 13 in]
            n118 = Select(t="DAQ: STOP\nDAQ: CLEAR\nMacro: Acquire" ("States Out"), s=w235, f=w231) -> (s? t:f=w230:string)
          }
          frame "Exit" {
            # "Do not put any code in this frame.\n(No errors that occur here will be handled.)"
            n119 = Unbundle By Name(w250) -> ("Core.error"=w249:errorcluster)
            n120 = call <vilib>:"Add State(s) to Queue__jki_lib_state_machine.vi"("State(s) in (\"\")"=w254) -> ("States Out"=w253:string)  [unwired: 14 in]
          }
          frame "---------- Data ----------" {
            # "Do not put any code in this frame.\n(It is a separator no-op. You can make a copy of this frame to create a new Data frame)"
            n121 = call <vilib>:"Add State(s) to Queue__jki_lib_state_machine.vi"("State(s) in (\"\")"=w259) -> ("States Out"=w258:string)  [unwired: 14 in]
          }
          frame "Data: Initialize" {
            w260 = dbl[] []  # Offset
            w261 = T6 {"Time Stamp"=timestamp(0 s since 1904-01-01), "X Results"=[], "Y Results"=[]}  # SweepResults []
            w262 = T6 {"Time Stamp"=timestamp(0 s since 1904-01-01), "X Results"=[], "Y Results"=[]}  # SweepResults [i]
            w263 = -1  # sweep index
            w264 = T7 10178 items=["Finite Samples"=10178, "Continuous Samples"=10123]  # sample mode
            w269 = T12 {"Time Stamp"=timestamp(0 s since 1904-01-01), "Results"=[]}  # Results
            w268 = State-enum."idle"  # state
            w271 = -1  # to
            w272 = waveform(dbl)[] []  # REF
            w274 = waveform(dbl)[] []  # AO
            w273 = waveform(dbl)[] []  # AI
            w275 = T27 {"Current VI Reference"=refnum, "Close Panel on Exit?"=FALSE, "error"={"status"=FALSE, "code"=0, "source"=""}}  # Core
            w278 = refnum<class "LockinDAQ.lvclass"> refnum  # Self Reference
            # "start in idle mode"
            # "do not delete - used by framework"
            # "Data names and types of shift register data are defined by this bundle."
            # "Initialize the shift-register data, here.\n(data names are defined by what you wire into the bundle function)"
            n122 = Variant To Data(error in=w279, type=w278, Variant=w277) -> (data=w267:refnum<class "LockinDAQ.lvclass">, error out=w266:errorcluster)
            n123 = call "LockinDAQ.getDAQState.vi"("error in (no error)"=w266, "state"=w268, "LockinDAQ"=w267) -> ("error out"=w265:errorcluster)  [unwired: 7 in, 1 out]
            n124 = local write "DAQ state"(w268) -> ()
            n125 = Bundle("Core"=w275, "Self Reference"=w267, "to"=w271, "state"=w268, "sample mode"=w264, "AO"=w274, "AI"=w273, "REF"=w272, "Results"=w269, "sweep index"=w263, "SweepResults [i]"=w262, "SweepResults []"=w261, "Offset"=w260) -> (w270:T13)  [unwired: 1 in]
            n126 = call <vilib>:"Add State(s) to Queue__jki_lib_state_machine.vi"("State(s) in (\"\")"=w281) -> ("States Out"=w280:string)  [unwired: 14 in]
          }
          frame "Data: Cleanup" {
            # "Cleanup any data and references, here.\n(this is called automatically, by the Macro: Exit)"
            n127 = Unbundle By Name(w283) -> ("Core.Current VI Reference"=w286:refnum<vi>)
            n128 = Close Reference(reference=w286, error in (no error)=w285) -> (error out=w284:errorcluster)
            n129 = call <vilib>:"Add State(s) to Queue__jki_lib_state_machine.vi"("State(s) in (\"\")"=w288) -> ("States Out"=w287:string)  [unwired: 14 in]
          }
          frame "---------- UI ----------" {
            # "Do not put any code in this frame.\n(It is a separator no-op. You can make a copy of this frame to create a new UI frame)"
            n130 = call <vilib>:"Add State(s) to Queue__jki_lib_state_machine.vi"("State(s) in (\"\")"=w293) -> ("States Out"=w292:string)  [unwired: 14 in]
          }
          frame "UI: Initialize" {
            # "Initialize the User Interface, here.\n(this is called automatically, by the Macro: Init)"
            n131 = local write "Method"("" ("String")) -> ()
            n132 = call <vilib>:"Add State(s) to Queue__jki_lib_state_machine.vi"("State(s) in (\"\")"=w299) -> ("States Out"=w298:string)  [unwired: 14 in]
          }
          frame "UI: Cursor Set" {
            # "Argument"
            # "Initialize the User Interface, here.\n(this is called automatically, by the Macro: Init)"
            n133 = disable-structure shown="Default" {
              disable-tunnel: w302 -> [w307 w310]
              disable-tunnel: [w307 w309] -> w301
              disable-tunnel: w300 -> [_ w308]
              frame condition #0 {
              }
              frame condition #1 (active) {
                n134 = case shown="\"Idle\", Default" w308 {
                  tunnel: w310 -> [w312 w314]
                  tunnel: [w311 w313] -> w309
                  frame "Idle", Default {
                    n135 = call <vilib>:"Unset Busy.vi"("error in (no error)"=w312) -> ("error out"=w311:errorcluster)  [unwired: 10 in]
                  }
                  frame "Busy" {
                    n136 = call <vilib>:"Set Busy.vi"("error in (no error)"=w314) -> ("error out"=w313:errorcluster)  [unwired: 9 in, 1 out]
                  }
                }
              }
            }
            n137 = call <vilib>:"Add State(s) to Queue__jki_lib_state_machine.vi"("State(s) in (\"\")"=w306) -> ("States Out"=w305:string)  [unwired: 14 in]
          }
          frame "UI: Front Panel State" {
            # "Argument"
            # "Set Front Panel Open or Closed\n(Usage: \"UI: Front Panel State >> Open|Close\")"
            n138 = Unbundle By Name(w318) -> ("Core.Current VI Reference"=w317:refnum<vi>)
            n139 = disable-structure shown="Default" {
              disable-tunnel: w320 -> [w326 w349]
              disable-tunnel: [w325 w349] -> w319
              disable-tunnel: w317 -> [w324 _]
              disable-tunnel: w316 -> [w323 _]
              frame condition #0 (active) {
                n140 = case shown="\"Close\"" w323 {
                  tunnel: w326 -> [w330 w343]
                  tunnel: [w332 w344] -> w325
                  tunnel: w324 -> [w331 w341]
                  frame "Open", Default {
                    n141 = property class="VI"(reference=w331, error in=w330) -> (reference out=w328:refnum<vi>, error out=w329:errorcluster, "FP.State"=w327:T4)
                    n142 = case shown="\"Closed\"" w327 {
                      tunnel: [w335 w338] -> w332
                      tunnel: w329 -> [w334 w338]
                      tunnel: w328 -> [w333 _]
                      frame "Closed" {
                        n143 = invoke class="VI" method="FP.Open"(reference=w333, error in=w334, "Activate"=TRUE, "State"=T4."Standard") -> (error out=w335:errorcluster)  [unwired: 1 in, 4 out]
                      }
                      frame Default {
                      }
                    }
                  }
                  frame "Close" {
                    n144 = property class="VI"(reference=w341, error in=w343) -> (reference out=w340:refnum<vi>, error out=w342:errorcluster, "FP.State"=w339:T4)
                    n145 = case shown="Default" w339 {
                      tunnel: [w345 w348] -> w344
                      tunnel: w342 -> [w345 w347]
                      tunnel: w340 -> [_ w346]
                      frame "Invalid", "Closed" {
                      }
                      frame Default {
                        n146 = invoke class="VI" method="FP.Close"(reference=w346, error in=w347) -> (error out=w348:errorcluster)  [unwired: 1 in, 2 out]
                      }
                    }
                  }
                }
              }
              frame condition #1 {
              }
            }
            n147 = call <vilib>:"Add State(s) to Queue__jki_lib_state_machine.vi"("State(s) in (\"\")"=w322) -> ("States Out"=w321:string)  [unwired: 14 in]
          }
          frame "---------- Macro ----------" {
            # "Do not put any code in this frame.\n(It is a separator no-op. You can make a copy of this frame to create a new Macro frame)"
            n148 = call <vilib>:"Add State(s) to Queue__jki_lib_state_machine.vi"("State(s) in (\"\")"=w354) -> ("States Out"=w353:string)  [unwired: 14 in]
          }
          frame "Macro: Initialize" {
            w359 = "UI: Initialize\nUI: Front Panel State >> Open"  # UI: Initialize UI: Front Panel State >> Open
            w355 = "Process: Sync"
            # "Initialization Macro\n(This is called once, when the VI starts)"
            n149 = control-ref of="This VI"() -> (w357:refnum<vi>)
            n150 = property class="VI"(reference=w357) -> ("Exec.State"=w356:T5)  [unwired: 1 in, 2 out]
            n151 = Equal?(x=w356, y=T5."Run top level") -> (x = y?=w362:bool)
            n152 = Select(t=w355, s=w362, f="") -> ()  [unwired: 1 out]
            n153 = call <vilib>:"Add State(s) to Queue__jki_lib_state_machine.vi"("State(s) in Front (\"\")"="Data: Initialize\nInitialize Core Data\nEvents: Register", "State(s) in (\"\")"=w355, "State(s) at Back (\"\")"=w359) -> ("States Out"=w358:string)  [unwired: 12 in]
            n154 = call <vilib>:"Add State(s) to Queue__jki_lib_state_machine.vi"("State(s) in Front (\"\")"=w358, "State(s) in (\"\")"=w368) -> ("States Out"=w367:string)  [unwired: 13 in]
          }
          frame "Macro: Exit" {
            # "Exit Macro\n(This is called once, when the VI exits)"
            n155 = Unbundle By Name(w374) -> ("Core.Close Panel on Exit?"=w379:bool)
            n156 = Select(t="UI: Front Panel State >> Close", s=w379, f="") -> (s? t:f=w376:string)
            n157 = call <vilib>:"Add State(s) to Queue__jki_lib_state_machine.vi"("State(s) in Front (\"\")"="Macro: Stop\nData: Cleanup\nEvents: Unregister", "State(s) in (\"\")"="Process: Sync", "State(s) at Back (\"\")"="Exit") -> ("States Out"=w371:string)  [unwired: 12 in]
            n158 = call <vilib>:"Add State(s) to Queue__jki_lib_state_machine.vi"("State(s) in (\"\")"=w376, "State(s) at Back (\"\")"=w371) -> ("States Out"=w369:string)  [unwired: 13 in]
            n159 = call <vilib>:"Add State(s) to Queue__jki_lib_state_machine.vi"("State(s) in Front (\"\")"=w369, "State(s) in (\"\")"=w382) -> ("States Out"=w381:string)  [unwired: 13 in]
          }
          frame "Macro: Acquire" {
            (unwired) "DAQ: TIMED LOOP\nDAQ: STOP\nDAQ: CLEAR" ("State(s) in Front (\"\")")
            w391 = 10178 items=["Finite Samples"=10178, "Continuous Samples"=10123] ("sample mode")
            # "#todo:\ndo not create/clear tasks every time"
            # "note (8/23/2019):\nCREATE/START & STOP/CLEAR go hand-in-hand in the macro, but they are separated to make it easier to add features (e.g. event registration b/w CREATE and START)"
            # "already running = \nDAQmx tasks are STARTED"
            n160 = Unbundle By Name(w390) -> ("state"=w384:T1, "sample mode"=w387:T7)
            n161 = Equal?(x=w387, y=w391) -> (x = y?=w386:bool)
            n162 = case shown="\"idle\", Default" w384 {
              tunnel: ["DAQ: CREATE\n//DAQ: Event\nDAQ: START" ("State(s) in Front (\"\")") "" ("State(s) in Front (\"\")")] -> w388
              frame "idle", Default {
              }
              frame "created" {
              }
            }
            n163 = case shown="True" w386 {
              tunnel: ["" ("State(s) in Front (\"\")") "DAQ: STOP\nDAQ: CLEAR" ("State(s) in Front (\"\")")] -> w385
              frame False {
              }
              frame True {
              }
            }
            n164 = call <vilib>:"Add State(s) to Queue__jki_lib_state_machine.vi"("State(s) in Front (\"\")"=w388, "State(s) in (\"\")"="Macro: Generate\nDAQ: AO AI\nMacro: DSP\nMacro: Sweep" ("State(s) in Front (\"\")"), "State(s) at Back (\"\")"=w385) -> ("States Out"=w389:string)  [unwired: 12 in]
            n165 = call <vilib>:"Add State(s) to Queue__jki_lib_state_machine.vi"("State(s) in Front (\"\")"=w389, "State(s) in (\"\")"=w395) -> ("States Out"=w394:string)  [unwired: 13 in]
          }
          frame "Macro: Generate" {
            # "Do not put any code in this frame.\n(It is a separator no-op. You can make a copy of this frame to create a new Macro frame)"
            n166 = call <vilib>:"Add State(s) to Queue__jki_lib_state_machine.vi"("State(s) in Front (\"\")"="Generate: Generate" ("State(s) in Front (\"\")"), "State(s) in (\"\")"=w405) -> ("States Out"=w404:string)  [unwired: 13 in]
          }
          frame "Macro: DSP" {
            # "Do not put any code in this frame.\n(It is a separator no-op. You can make a copy of this frame to create a new Macro frame)"
            n167 = call <vilib>:"Add State(s) to Queue__jki_lib_state_machine.vi"("State(s) in Front (\"\")"="DSP: Phase" ("State(s) in Front (\"\")"), "State(s) at Back (\"\")"="DSP: Filter\nDSP: Lockin" ("State(s) in Front (\"\")")) -> ("States Out"=w408:string)  [unwired: 13 in]
            n168 = call <vilib>:"Add State(s) to Queue__jki_lib_state_machine.vi"("State(s) in Front (\"\")"=w408, "State(s) in (\"\")"=w413) -> ("States Out"=w412:string)  [unwired: 13 in]
          }
          frame "Macro: Sweep" {
            n169 = Unbundle By Name(w418) -> ("Self Reference"=w417:refnum<class "LockinDAQ.lvclass">, "sweep index"=w416:i32)
            n170 = case shown="4" w416 {
              tunnel: ["" ("State(s) in Front (\"\")") "Sweep: Initialize\nSweep: Set Initial\nSweep: Wait" ("State(s) in Front (\"\")") "Sweep: Wait" ("State(s) in Front (\"\")") "Sweep: Configure Sweep" ("State(s) in Front (\"\")") "Sweep: Save\nSweep: Done Sweeping?" ("State(s) in Front (\"\")") "Sweep: Stop" ("State(s) in Front (\"\")")] -> w415
              tunnel: w417 -> [_ _ _ _ _ _]
              frame -1, Default {
              }
              frame 0 {
              }
              frame 1 {
              }
              frame 2 {
              }
              frame 3 {
              }
              frame 4 {
              }
            }
            n171 = call <vilib>:"Add State(s) to Queue__jki_lib_state_machine.vi"("State(s) in Front (\"\")"=w415, "State(s) in (\"\")"=w421) -> ("States Out"=w420:string)  [unwired: 13 in]
          }
          frame "Macro: Stop" {
            n172 = call <vilib>:"Add State(s) to Queue__jki_lib_state_machine.vi"("State(s) in Front (\"\")"="DAQ: STOP\nDAQ: CLEAR" ("State(s) in Front (\"\")"), "State(s) in (\"\")"=w433) -> ("States Out"=w429:string)  [unwired: 13 in]
          }
          frame "---------- Process ----------" {
            # "Template Separator\n(You can make a copy of, or modify, this frame)"
            n173 = call <vilib>:"Add State(s) to Queue__jki_lib_state_machine.vi"("State(s) in (\"\")"=w438) -> ("States Out"=w437:string)  [unwired: 14 in]
          }
          frame "Process: Sync" {
            n174 = Unbundle By Name(w446) -> ("Self Reference"=w442:refnum<class "LockinDAQ.lvclass">)
            n175 = call <vilib>:"WaitOnProcessSync.vi"("error in (no error)"=w441, "SMO"=w442) -> ("error out"=w440:errorcluster, "Don't run?"=w445:bool)  [unwired: 7 in, 1 out]
            n176 = Select(t="Data: Cleanup\nEvents: Unregister\nExit", s=w445, f="") -> (s? t:f=w439:string)
            n177 = call <vilib>:"Add State(s) to Queue__jki_lib_state_machine.vi"("State(s) in Front (\"\")"=w439, "State(s) in (\"\")"=w449) -> ("States Out"=w448:string)  [unwired: 13 in]
          }
          frame "---------- Events ----------" {
            # "Template Separator\n(You can make a copy of, or modify, this frame)"
            n178 = call <vilib>:"Add State(s) to Queue__jki_lib_state_machine.vi"("State(s) in (\"\")"=w454) -> ("States Out"=w453:string)  [unwired: 14 in]
          }
          frame "Events: Register" {
            w455 = refnum<event-registration> refnum  # DAQmx
            w463 = refnum<event-registration> refnum  # SMO
            w464 = refnum<event-registration> refnum  # LockinDAQ
            # "Replace later"
            # "Expand to add\nmore events"
            n179 = Unbundle By Name(w475) -> ("Self Reference"=w474:refnum<class "LockinDAQ.lvclass">)
            n180 = call <vilib>:"GetProtectedEvents.vi"("SMO"=w474) -> ("error out"=w471:errorcluster, "SMO Protected Events"=w467:T28, "SMO out"=w470:refnum<class "LockinDAQ.lvclass">)  [unwired: 8 in]
            n181 = call "LockinDAQ.GetPrivateEvents.vi"("LockinDAQ"=w470) -> ("error out"=w457:errorcluster, "Private Events"=w466:T29)  [unwired: 8 in, 1 out]
            n182 = register-events(w467) -> (reference out=w469:refnum<event-registration>, error out=w462:errorcluster)  [unwired: 2 in]
            n183 = register-events(w466) -> (reference out=w465:refnum<event-registration>, error out=w459:errorcluster)  [unwired: 2 in]
            n184 = Variant To Data(error in=w459, type=w464, Variant=w465) -> (data=w456:refnum<event-registration>, error out=w460:errorcluster)
            n185 = Variant To Data(error in=w462, type=w463, Variant=w469) -> (data=w458:refnum<event-registration>, error out=w461:errorcluster)
            n186 = Bundle("SMO"=w458, "LockinDAQ"=w456, "DAQmx"=w455) -> (w468:T30)  [unwired: 1 in]
            n187 = Merge Errors(w461, w460, w457, w473, w471) -> (w472:errorcluster)
            n188 = call <vilib>:"Add State(s) to Queue__jki_lib_state_machine.vi"("State(s) in (\"\")"=w477) -> ("States Out"=w476:string)  [unwired: 14 in]
          }
          frame "Events: Unregister" {
            n189 = Unregister For Events(event registration refnum=w478, error in=w480) -> (error out=w479:errorcluster)
            n190 = call <vilib>:"Clear Errors.vi"("error in (no error)"=w479) -> ()  [unwired: 5 in, 2 out]
            n191 = call <vilib>:"Add State(s) to Queue__jki_lib_state_machine.vi"("State(s) in (\"\")"=w483) -> ("States Out"=w482:string)  [unwired: 14 in]
          }
          frame "---------- DAQ ----------" {
            n192 = call <vilib>:"Add State(s) to Queue__jki_lib_state_machine.vi"("State(s) in (\"\")"=w488) -> ("States Out"=w487:string)  [unwired: 14 in]
          }
          frame "DAQ: CREATE" {
            n193 = Unbundle By Name(w502) -> ("Self Reference"=w500:refnum<class "LockinDAQ.lvclass">, "state"=w490:T1)
            n194 = call <userlib>:"Tick Count (ms)__ogtk.vi"("error in (no error)"=w499) -> ("error out"=w493:errorcluster, "millisecond timer value"=w496:u32)  [unwired: 9 in]
            n195 = case shown="\"idle\"" w490 {
              selector: w490 -> [w509 _]
              tunnel: w500 -> [w508 w519]
              tunnel: [w508 w512] -> w494
              tunnel: w493 -> [w507 w518]
              tunnel: [w507 w513] -> w492
              tunnel: [w509 w511] -> w491
              tunnel: ["" ("State(s) in Front (\"\")") w510] -> w489
              frame Default {
              }
              frame "idle" {
                # "create DAQ tasks"
                n196 = call "LockinDAQ.Create.vi"("error in"=w518, "LockinDAQ"=w519) -> ("error out"=w515:errorcluster, "LockinDAQ out"=w514:refnum<class "LockinDAQ.lvclass">)  [unwired: 8 in]
                n197 = case shown="No Error" w515 {
                  selector: w515 -> [w522 w526]
                  tunnel: [State-enum."created" ("state") State-enum."idle" ("state")] -> w511
                  tunnel: [w522 w526] -> w516
                  tunnel: w514 -> [w521 w525]
                  tunnel: [w521 w525] -> w517
                  tunnel: ["" ("State(s) in Front (\"\")") "DAQ: CLEAR" ("State(s) in Front (\"\")")] -> w510
                  frame No Error {
                  }
                  frame Error {
                  }
                }
                n198 = call "LockinDAQ.getDAQState.vi"("error in (no error)"=w516, "state"=w511, "LockinDAQ"=w517) -> ("error out"=w513:errorcluster, "LockinDAQ out"=w512:refnum<class "LockinDAQ.lvclass">)  [unwired: 7 in]
              }
            }
            n199 = Bundle By Name(cluster=w502, "Self Reference"=w494, "state"=w491) -> (w501:T13)
            n200 = local write "DAQ state"(w491) -> ()
            n201 = call <userlib>:"Tick Count (ms)__ogtk.vi"("error in (no error)"=w492) -> ("error out"=w498:errorcluster, "millisecond timer value"=w497:u32)  [unwired: 9 in]
            n202 = Subtract(x=w497, y=w496) -> (x-y=→"DAQ Create Tasks (ms)":u32)
            n203 = call <vilib>:"Add State(s) to Queue__jki_lib_state_machine.vi"("State(s) in Front (\"\")"=w489, "State(s) in (\"\")"=w505) -> ("States Out"=w504:string)  [unwired: 13 in]
          }
          frame "DAQ: START" {
            n204 = Unbundle By Name(w542) -> ("to"=w528:i32, "Self Reference"=w540:refnum<class "LockinDAQ.lvclass">, "state"=w529:T1)
            n205 = call <userlib>:"Tick Count (ms)__ogtk.vi"("error in (no error)"=w539) -> ("error out"=w534:errorcluster, "millisecond timer value"=w536:u32)  [unwired: 9 in]
            n206 = case shown="\"started\", \"sweeping\"" w529 {
              selector: w529 -> [_ w566]
              tunnel: w540 -> [w555 w565]
              tunnel: w534 -> [w551 w567]
              tunnel: [w550 w567] -> w533
              tunnel: [w548 w565] -> w532
              tunnel: [w547 w564] -> w531
              tunnel: [w546 w566] -> w530
              tunnel: w528 -> [_ w564]
              frame Default {
                n207 = call "LockinDAQ.Start.vi"("error in"=w551, "LockinDAQ"=w555) -> ("error out"=w554:errorcluster, "LockinDAQ out"=w552:refnum<class "LockinDAQ.lvclass">)  [unwired: 8 in]
                n208 = case shown="No Error" w554 {
                  selector: w554 -> [w557 w561]
                  tunnel: [State-enum."started" ("state") State-enum."idle" ("state")] -> w546
                  tunnel: [1 -1] -> w547
                  tunnel: [w557 w561] -> w553
                  tunnel: w552 -> [w556 w560]
                  tunnel: [w556 w560] -> w549
                  frame No Error {
                  }
                  frame Error {
                  }
                }
                n209 = call "LockinDAQ.getDAQState.vi"("error in (no error)"=w553, "state"=w546, "LockinDAQ"=w549) -> ("error out"=w550:errorcluster, "LockinDAQ out"=w548:refnum<class "LockinDAQ.lvclass">)  [unwired: 7 in]
              }
              frame "started", "sweeping" {
              }
            }
            "DAQ state" <- w530
            n210 = Bundle By Name(cluster=w542, "to"=w531, "Self Reference"=w532, "state"=w530) -> (w541:T13)
            n211 = call <userlib>:"Tick Count (ms)__ogtk.vi"("error in (no error)"=w533) -> ("error out"=w538:errorcluster, "millisecond timer value"=w537:u32)  [unwired: 9 in]
            n212 = Subtract(x=w537, y=w536) -> (x-y=→"DAQ Start Tasks (ms)":u32)
            n213 = call <vilib>:"Add State(s) to Queue__jki_lib_state_machine.vi"("State(s) in (\"\")"=w545) -> ("States Out"=w544:string)  [unwired: 14 in]
          }
          frame "DAQ: AO AI" {
            # "write AO\nread AI"
            n214 = call <userlib>:"Tick Count (ms)__ogtk.vi"("error in (no error)"=w578) -> ("error out"=w573:errorcluster, "millisecond timer value"=w570:u32)  [unwired: 9 in]
            n215 = Unbundle By Name(w580) -> ("Self Reference"=w577:refnum<class "LockinDAQ.lvclass">, "AO"=w576:waveform(dbl)[])
            n216 = call "LockinDAQ.Read AI and Write AO.vi"("error in (no error)"=w573, "AO []"=w576, "LockinDAQ"=w577) -> ("error out"=w574:errorcluster, "AI []"=w568:waveform(dbl)[], "LockinDAQ out"=w575:refnum<class "LockinDAQ.lvclass">)  [unwired: 6 in]
            n217 = Bundle By Name(cluster=w580, "Self Reference"=w575, "AI"=w568) -> (w579:T13)
            n218 = call <userlib>:"Tick Count (ms)__ogtk.vi"("error in (no error)"=w574) -> ("error out"=w572:errorcluster, "millisecond timer value"=w571:u32)  [unwired: 9 in]
            n219 = Subtract(x=w571, y=w570) -> (x-y=→"DAQ AO/AI (ms)":u32)
            n220 = call <vilib>:"Add State(s) to Queue__jki_lib_state_machine.vi"("State(s) in (\"\")"=w583) -> ("States Out"=w582:string)  [unwired: 14 in]
          }
          frame "DAQ: TIMED LOOP" {
            # "!!!!!!!!!!!!!!!!!!!!!!!!!!!!!!!!!!!!!!!!!!!!!!!!!!!!!!!!!!!!!!!!!!!!!!!!\nTHIS IS AN EXPERIMENTAL BLOCKING CALL TO:\nGenerate\nRead/Write\nDSP\nIt should listen to events that change AO or REF Channels.\nInside there is a timed loop that will not stop unless it receives events for Set State = stop; SMO Stop; or SMO error\n!!!!!!!!!!!!!!!!!!!!!!!!!!!!!!!!!!!!!!!!!!!!!!!!!!!!!!!!!!!!!!!!!!!!!"
            n221 = Unbundle By Name(w590) -> ("Self Reference"=w587:refnum<class "LockinDAQ.lvclass">)
            n222 = call "LockinDAQ.TimedLoop.vi"("error in (no error)"=w585, "Event Cluster"=w588, "LockinDAQ"=w587) -> ("error out"=w584:errorcluster, "SMO out"=w586:refnum<class "LockinDAQ.lvclass">)  [unwired: 7 in]
            n223 = Bundle By Name(cluster=w590, "Self Reference"=w586) -> (w589:T13)
            n224 = call <vilib>:"Add State(s) to Queue__jki_lib_state_machine.vi"("State(s) in (\"\")"=w592) -> ("States Out"=w591:string)  [unwired: 14 in]
          }
          frame "DAQ: CALIBRATE" {
            # "calibrate or get calibration"
            n225 = Unbundle By Name(w599) -> ("Self Reference"=w596:refnum<class "LockinDAQ.lvclass">)
            n226 = case shown="\"False\", Default" w597 {
              tunnel: w596 -> [w606 w610]
              tunnel: [w605 w609] -> w595
              tunnel: w594 -> [w603 w608]
              tunnel: [w604 w607] -> w593
              frame "False", Default {
                n227 = call "LockinDAQ.Get Calibration.vi"("error in (no error)"=w603, "LockinDAQ"=w606) -> ("error out"=w604:errorcluster, "LockinDAQ out"=w605:refnum<class "LockinDAQ.lvclass">)  [unwired: 7 in, 1 out]
              }
              frame "True" {
                n228 = call "LockinDAQ.Calibrate.vi"("error in (no error)"=w608, "LockinDAQ"=w610) -> ("error out"=w607:errorcluster, "LockinDAQ out"=w609:refnum<class "LockinDAQ.lvclass">)  [unwired: 7 in, 1 out]
              }
            }
            n229 = Bundle By Name(cluster=w599, "Self Reference"=w595) -> (w598:T13)
            n230 = call <vilib>:"Add State(s) to Queue__jki_lib_state_machine.vi"("State(s) in (\"\")"=w602) -> ("States Out"=w601:string)  [unwired: 14 in]
          }
          frame "DAQ: STOP" {
            n231 = Unbundle By Name(w620) -> ("to"=w613:i32, "Self Reference"=w618:refnum<class "LockinDAQ.lvclass">, "state"=w616:T1)
            n232 = case shown="Default" w616 {
              selector: w616 -> [w625 w629]
              tunnel: w618 -> [w627 w637]
              tunnel: w617 -> [w624 w636]
              tunnel: [w627 w630] -> w615
              tunnel: [w626 w633] -> w614
              tunnel: w613 -> [w626 w628]
              tunnel: [w624 w632] -> w612
              tunnel: [w625 w631] -> w611
              frame "idle", "stopped" {
              }
              frame Default {
                # "stop DAQmx tasks"
                n233 = call "LockinDAQ.Stop.vi"("error in (no error)"=w636, "LockinDAQ"=w637) -> ("error out"=w635:errorcluster, "LockinDAQ out"=w634:refnum<class "LockinDAQ.lvclass">)  [unwired: 8 in]
                n234 = case shown="No Error" w635 {
                  selector: w635 -> [w641 w644]
                  tunnel: w634 -> [w642 w645]
                  tunnel: [-1 ("to") w646] -> w633
                  tunnel: [w640 w644] -> w632
                  tunnel: [w639 w647] -> w631
                  tunnel: [w638 w645] -> w630
                  tunnel: w629 -> [_ w647]
                  tunnel: w628 -> [_ w646]
                  frame No Error {
                    w639 = State-enum."stopped" ("state")
                    n235 = call "LockinDAQ.getDAQState.vi"("error in (no error)"=w641, "state"=w639, "LockinDAQ"=w642) -> ("error out"=w640:errorcluster, "LockinDAQ out"=w638:refnum<class "LockinDAQ.lvclass">)  [unwired: 7 in]
                  }
                  frame Error {
                  }
                }
              }
            }
            n236 = Bundle By Name(cluster=w620, "to"=w614, "Self Reference"=w615, "state"=w611) -> (w619:T13)
            n237 = local write "DAQ state"(w611) -> ()
            n238 = call <vilib>:"Add State(s) to Queue__jki_lib_state_machine.vi"("State(s) in (\"\")"=w623) -> ("States Out"=w622:string)  [unwired: 14 in]
          }
          frame "DAQ: CLEAR" {
            w649 = State-enum."idle" ("state")
            # "clear DAQmx tasks"
            n239 = Unbundle By Name(w657) -> ("Self Reference"=w655:refnum<class "LockinDAQ.lvclass">)
            n240 = call "LockinDAQ.Clear.vi"("error in (no error)"=w654, "LockinDAQ"=w655) -> ("error out"=w653:errorcluster, "LockinDAQ out"=w652:refnum<class "LockinDAQ.lvclass">)  [unwired: 8 in]
            n241 = call "LockinDAQ.getDAQState.vi"("error in (no error)"=w653, "state"=w649, "LockinDAQ"=w652) -> ("error out"=w648:errorcluster, "LockinDAQ out"=w650:refnum<class "LockinDAQ.lvclass">)  [unwired: 7 in]
            n242 = Bundle By Name(cluster=w657, "to"=-1, "Self Reference"=w650, "state"=w649) -> (w656:T13)
            n243 = local write "DAQ state"(w649) -> ()
            n244 = call <vilib>:"Add State(s) to Queue__jki_lib_state_machine.vi"("State(s) in (\"\")"=w660) -> ("States Out"=w659:string)  [unwired: 14 in]
          }
          frame "DAQ: Event" {
            # "Experimental state: generates a user event\nwhen there are a sufficient number of samples.\nUse to drive sequence instead of timeout"
            n245 = Unbundle By Name(w668) -> ("DAQmx"=w667:refnum<event-registration>)
            n246 = Unbundle By Name(w663) -> ("Self Reference"=w670:refnum<class "LockinDAQ.lvclass">)
            n247 = call "LockinDAQ.EventRegistration.vi"("error in (no error)"=w665, "DAQmx in"=w667, "LockinDAQ in"=w670) -> ("error out"=w664:errorcluster, "DAQmx out"=w666:refnum<event-registration>, "LockinDAQ out"=w661:refnum<class "LockinDAQ.lvclass">)  [unwired: 6 in]
            n248 = Bundle By Name(cluster=w663, "Self Reference"=w661) -> (w662:T13)
            n249 = Bundle By Name(cluster=w668, "DAQmx"=w666) -> (w669:T30)
            n250 = call <vilib>:"Add State(s) to Queue__jki_lib_state_machine.vi"("State(s) in (\"\")"=w672) -> ("States Out"=w671:string)  [unwired: 14 in]
          }
          frame "---------- DSP ----------" {
            n251 = call <vilib>:"Add State(s) to Queue__jki_lib_state_machine.vi"("State(s) in (\"\")"=w677) -> ("States Out"=w676:string)  [unwired: 14 in]
          }
          frame "DSP: Phase" {
            # "PRIVATE"
            # "PRIVATE"
            # "PRIVATE"
            # "PRIVATE"
            # "PRIVATE"
            n252 = Unbundle By Name(w682) -> ("Results"=w684:T12, "Self Reference"=w683:refnum<class "LockinDAQ.lvclass">)
            n253 = call "lockin - add phase element.vi"("error in (no error)"=w680, "LockinDAQ"=w683) -> ("error out"=w691:errorcluster, "LockinDAQ out"=w692:refnum<class "LockinDAQ.lvclass">)  [unwired: 8 in]
            n254 = case shown="True" "reset REF" {
              tunnel: w691 -> [w697 w701]
              tunnel: w692 -> [w696 w700]
              tunnel: [w697 w699] -> w689
              tunnel: [w696 w698] -> w688
              frame False {
              }
              frame True {
                n255 = call "lockin - Set REF phase equals zero.vi"("error in (no error)"=w701, "LockinDAQ out"=w700) -> ("error out"=w699:errorcluster, "LockinDAQ"=w698:refnum<class "LockinDAQ.lvclass">)  [unwired: 8 in]
              }
            }
            n256 = case shown="True" "autophase?\n(experimental)" {
              tunnel: w684 -> [_ w708]
              tunnel: w689 -> [w703 w707]
              tunnel: w688 -> [w702 w706]
              tunnel: [w703 w705] -> w687
              tunnel: [w702 w704] -> w685
              frame False {
              }
              frame True {
                n257 = call "4461 Autophase.vi"("error in (no error)"=w707, "Results"=w708, "LockinDAQ"=w706) -> ("error out"=w705:errorcluster, "LockinDAQ out"=w704:refnum<class "LockinDAQ.lvclass">)  [unwired: 7 in]
              }
            }
            n258 = call "4461 Replace AO Ch.vi"("error in (no error)"=w687, "LockinDAQ (NEW)"=w685, "LockinDAQ (OLD)"=w683) -> ("error out"=w679:errorcluster, "LockinDAQ out"=w678:refnum<class "LockinDAQ.lvclass">)  [unwired: 7 in]
            n259 = Bundle By Name(cluster=w682, "Self Reference"=w678) -> (w681:T13)
            n260 = call <vilib>:"Add State(s) to Queue__jki_lib_state_machine.vi"("State(s) in (\"\")"=w695) -> ("States Out"=w694:string)  [unwired: 14 in]
          }
          frame "DSP: Filter" {
            w717 = 1  # decimating factor
            w716 = FALSE  # averaging
            # "publish AI waveform"
            n261 = Unbundle By Name(w735) -> ("Self Reference"=w713:refnum<class "LockinDAQ.lvclass">, "AO"=w714:waveform(dbl)[], "REF"=w715:waveform(dbl)[], "AI"=w710:waveform(dbl)[], "Offset"=w709:dbl[])
            n262 = call "decimate_waveforms.vi"("decimating factor"=w717, "averaging"=w716, "error in (no error)"=w723, "WFM"=w714) -> ("error out"=w729:errorcluster, "WFM out"=w720:waveform(dbl)[])  [unwired: 6 in]
            n263 = call "decimate_waveforms.vi"("decimating factor"=w717, "averaging"=w716, "error in (no error)"=w723, "WFM"=w715) -> ("error out"=w730:errorcluster, "WFM out"=w721:waveform(dbl)[])  [unwired: 6 in]
            n264 = call "decimate_waveforms.vi"("decimating factor"=w717, "averaging"=w716, "error in (no error)"=w723, "WFM"=w710) -> ("error out"=w726:errorcluster, "WFM out"=w718:waveform(dbl)[])  [unwired: 6 in]
            n265 = Merge Errors(w729, w730, w726) -> (w712:errorcluster)
            n266 = call "Subtract Offset.vi"("error in (no error)"=w712, "Offset"=w709, "WFM in"=w718) -> ("error out"=w722:errorcluster, "WFM out"=w719:waveform(dbl)[])  [unwired: 7 in]
            n267 = case shown="True" "60 Hz Prefilter?" {
              tunnel: w719 -> [w747 w751]
              tunnel: [w747 w750] -> w732
              tunnel: w722 -> [w746 w749]
              tunnel: [w746 w748] -> w731
              frame False {
              }
              frame True {
                n268 = call "Prefilter_60Hz_Notch.vi"("error in (no error)"=w749, "Array in"=w751) -> ("error out"=w748:errorcluster, "Array out"=w750:waveform(dbl)[])  [unwired: 8 in]
              }
            }
            n269 = case shown="True" "LP filter?" {
              tunnel: w732 -> [w740 w745]
              tunnel: [w740 w741] -> w728
              tunnel: w731 -> [w739 w743]
              tunnel: [w739 w742] -> w711
              tunnel: "LP Cutoff (Hz)" -> [_ w744]
              frame False {
              }
              frame True {
                n270 = call "Prefilter_LP.vi"("error in (no error)"=w743, "high cutoff freq [Hz]"=w744, "WFM in"=w745) -> ("error out"=w742:errorcluster, "WFM out"=w741:waveform(dbl)[])  [unwired: 7 in]
              }
            }
            n271 = Bundle By Name(cluster=w735, "AO"=w720, "REF"=w721, "AI"=w728) -> (w734:T13)
            n272 = call "LockinDAQ.getAI.vi"("error in (no error)"=w711, "getAI"=w728, "LockinDAQ"=w713) -> ("error out"=w727:errorcluster)  [unwired: 7 in, 1 out]
            n273 = call <vilib>:"Add State(s) to Queue__jki_lib_state_machine.vi"("State(s) in (\"\")"=w738) -> ("States Out"=w737:string)  [unwired: 14 in]
          }
          frame "DSP: Lockin" {
            # "publish Results"
            # "lockin demodulation"
            n274 = Unbundle By Name(w771) -> ("Self Reference"=w754:refnum<class "LockinDAQ.lvclass">, "AI"=w756:waveform(dbl)[], "REF"=w752:waveform(dbl)[])
            n275 = call <userlib>:"Tick Count (ms)__ogtk.vi"("error in (no error)"=w769) -> ("error out"=w758:errorcluster, "millisecond timer value"=w761:u32)  [unwired: 9 in]
            n276 = call "Divide Gain.vi"("error in (no error)"=w758, "WFM in"=w756, "LockinDAQ"=w754) -> ("error out"=w757:errorcluster, "WFM out"=w759:waveform(dbl)[], "LockinDAQ out"=w753:refnum<class "LockinDAQ.lvclass">)  [unwired: 6 in]
            n277 = call "Lockin Engine.vi"("error in (no error)"=w757, "REF Waveforms"=w752, "AI Waveforms"=w759, "LockinDAQ"=w753) -> ("error out"=w765:errorcluster, "SweepResults"=w755:T6, "Averaged Results (X,Y,R,Theta,Mean)"=w766:T12, "LockinDAQ out"=w768:refnum<class "LockinDAQ.lvclass">)  [unwired: 4 in]
            n278 = call "LockinDAQ.getResults.vi"("error in (no error)"=w765, "Results"=w766, "LockinDAQ"=w768) -> ("error out"=w764:errorcluster, "LockinDAQ out"=w767:refnum<class "LockinDAQ.lvclass">)  [unwired: 7 in]
            n279 = Bundle By Name(cluster=w771, "Self Reference"=w767, "Results"=w766, "SweepResults [i]"=w755) -> (w770:T13)
            n280 = call <userlib>:"Tick Count (ms)__ogtk.vi"("error in (no error)"=w764) -> ("error out"=w763:errorcluster, "millisecond timer value"=w762:u32)  [unwired: 9 in]
            n281 = Subtract(x=w762, y=w761) -> (x-y=→"Lockin (ms)":u32)
            n282 = call <vilib>:"Add State(s) to Queue__jki_lib_state_machine.vi"("State(s) in (\"\")"=w774) -> ("States Out"=w773:string)  [unwired: 14 in]
          }
          frame "DSP: Measure Offset" {
            # "remove any existing offset\nbefore calculating new offset"
            # "reset indicator after measuring"
            n283 = Unbundle By Name(w786) -> ("AI"=w775:waveform(dbl)[], "Offset"=w780:dbl[])
            n284 = Negate(x=w780) -> (-x=w779:dbl[])
            n285 = call "Subtract Offset.vi"("error in (no error)"=w777, "Offset"=w779, "WFM in"=w775) -> ("error out"=w776:errorcluster, "WFM out"=w778:waveform(dbl)[])  [unwired: 7 in]
            n286 = call-poly <vilib>:"Basic Averaged DC-RMS.vi"("reset"=TRUE, "error in (no error)"=w776, "signals in"=w778) -> ("error out"=w782:errorcluster, "DC values"=w784:dbl[])  [unwired: 5 in, 2 out]
            n287 = Bundle By Name(cluster=w786, "Offset"=w784) -> (w785:T13)
            n288 = local write "measure offset"(FALSE ("measureOffset")) -> ()
            n289 = call <vilib>:"Add State(s) to Queue__jki_lib_state_machine.vi"("State(s) in (\"\")"=w789) -> ("States Out"=w788:string)  [unwired: 14 in]
          }
          frame "DSP: Remove Offset" {
            # "reset indicator after zeroing"
            n290 = Unbundle By Name(w792) -> ("AI"=w791:waveform(dbl)[])
            n291 = for {
              tunnel: w791 -> [_] mode=indexing
              tunnel: [0.0] -> w790 mode=indexing
            }
            n292 = local write "zero offset"(FALSE ("measureOffset")) -> ()
            n293 = Bundle By Name(cluster=w792, "Offset"=w790) -> (w794:T13)
            n294 = call <vilib>:"Add State(s) to Queue__jki_lib_state_machine.vi"("State(s) in (\"\")"=w798) -> ("States Out"=w797:string)  [unwired: 14 in]
          }
          frame "---------- Sweep ----------" {
            n295 = call <vilib>:"Add State(s) to Queue__jki_lib_state_machine.vi"("State(s) in (\"\")"=w804) -> ("States Out"=w803:string)  [unwired: 14 in]
          }
          frame "Sweep: Initialize" {
            w813 = State-enum."sweeping" ("state")
            n296 = Unbundle By Name(w816) -> ("Self Reference"=w809:refnum<class "LockinDAQ.lvclass">)
            n297 = Unbundle By Name(w809) -> ("Channels: AO"=w808:T18)
            n298 = Bundle By Name(cluster=w809, "Saved Channels: AO"=w808) -> (w811:refnum<class "LockinDAQ.lvclass">)
            n299 = Get Date/Time In Seconds() -> (seconds since 1Jan1904=w806:timestamp)
            n300 = Bundle By Name(cluster=T6 {"Time Stamp"=timestamp(0 s since 1904-01-01), "X Results"=[], "Y Results"=[]} ("All Results []"), "Time Stamp"=w806) -> (w805:T6)
            n301 = Bundle By Name(cluster=w816, "Self Reference"=w811, "SweepResults []"=w805, "state"=w813, "sweep index"=0) -> (w815:T13)
            n302 = call "LockinDAQ.getDAQState.vi"("error in (no error)"=w810, "state"=w813, "LockinDAQ"=w811) -> ("error out"=w814:errorcluster)  [unwired: 7 in, 1 out]
            n303 = call <vilib>:"Add State(s) to Queue__jki_lib_state_machine.vi"("State(s) in (\"\")"=w819) -> ("States Out"=w818:string)  [unwired: 14 in]
          }
          frame "Sweep: Set Initial" {
            # "1: Set Initial Vstart"
            n304 = Unbundle By Name(w825) -> ("Self Reference"=w821:refnum<class "LockinDAQ.lvclass">)
            n305 = call "LockinDAQ.Set Initial Value.vi"("error in (no error)"=w823, "LockinDAQ in"=w821) -> ("error out"=w820:errorcluster, "LockinDAQ out"=w822:refnum<class "LockinDAQ.lvclass">)  [unwired: 8 in]
            n306 = Bundle By Name(cluster=w825, "Self Reference"=w822) -> (w824:T13)
            n307 = call <vilib>:"Add State(s) to Queue__jki_lib_state_machine.vi"("State(s) in (\"\")"=w828) -> ("States Out"=w827:string)  [unwired: 14 in]
          }
          frame "Sweep: Wait" {
            n308 = Unbundle By Name(w831) -> ("sweep index"=w836:i32, "Self Reference"=w829:refnum<class "LockinDAQ.lvclass">)
            n309 = Unbundle By Name(w829) -> ("Initial Wait Time (s)"=w837:dbl)
            n310 = Equal To 0?(x=w836) -> (x = 0?=w835:bool)
            n311 = Multiply(x=w837, y=1000.0) -> (x*y=w833:dbl)
            n312 = call <userlib>:"Periodic Trigger__ogtk.vi"("time (ms)"=w833, "reset"=w835) -> ("Triggered"=w834:bool)  [unwired: 11 in, 2 out]
            n313 = case shown="True" w834 {
              tunnel: [1 ("sweep index") 2 ("sweep index")] -> w832
              frame False {
              }
              frame True {
              }
            }
            n314 = Bundle By Name(cluster=w831, "sweep index"=w832) -> (w830:T13)
            n315 = call <vilib>:"Add State(s) to Queue__jki_lib_state_machine.vi"("State(s) in (\"\")"=w842) -> ("States Out"=w841:string)  [unwired: 14 in]
          }
          frame "Sweep: Configure Sweep" {
            # "2. Setup Sweep from Vstart to Vend in Time_sweep"
            n316 = Unbundle By Name(w851) -> ("Self Reference"=w849:refnum<class "LockinDAQ.lvclass">)
            n317 = call "LockinDAQ.Configure Sweep.vi"("error in (no error)"=w848, "LockinDAQ in"=w849) -> ("error out"=w846:errorcluster, "LockinDAQ out"=w847:refnum<class "LockinDAQ.lvclass">)  [unwired: 8 in]
            n318 = Bundle By Name(cluster=w851, "Self Reference"=w847, "sweep index"=3) -> (w850:T13)
            n319 = call <vilib>:"Add State(s) to Queue__jki_lib_state_machine.vi"("State(s) in (\"\")"=w854) -> ("States Out"=w853:string)  [unwired: 14 in]
          }
          frame "Sweep: Done Sweeping?" {
            # "#todo\ndo something more sophisticated...like compate 1st and last points of array\nand decide if next write will be more"
            # "within 0.010% of last point?"
            # "get last point"
            n320 = Unbundle By Name(w859) -> ("AO"=w862:waveform(dbl)[], "Self Reference"=w855:refnum<class "LockinDAQ.lvclass">)
            n321 = Unbundle By Name(w855) -> ("Sweep Channel"=w857:i32[], "Sweep End (V)"=w856:dbl[])
            n322 = Decrement(x=w857) -> (x-1=w868:i32[])
            n323 = Index Array(array=w862, index=w868) -> (element=w869:waveform(dbl))
            n324 = Unbundle By Name(w869) -> ("Y"=w867:dbl[])
            n325 = Reverse 1D Array(array=w867) -> (reversed array=w866:dbl[])
            n326 = Index Array(array=w866) -> (element=w861:dbl)  [unwired: 1 in]
            n327 = Divide(x=w861, y=w856) -> (x/y=w863:dbl[])
            n328 = In Range and Coerce(upper limit=1.0001, x=w863, lower limit=0.9999 ("upper limit")) -> (In Range?=w860:bool[])  [unwired: 1 out]
            n329 = case shown="False" w860 {
              tunnel: w859 -> [w874 w877]
              tunnel: [w874 w876] -> w858
              frame False {
              }
              frame True {
                n330 = Bundle By Name(cluster=w877, "sweep index"=4) -> (w876:T13)
              }
            }
            n331 = call <vilib>:"Add State(s) to Queue__jki_lib_state_machine.vi"("State(s) in (\"\")"=w873) -> ("States Out"=w872:string)  [unwired: 14 in]
          }
          frame "Sweep: Save" {
            # "this one needs to be more dynamic in case we are sweeping f or phase"
            # "Gather most recent results array and add to previous results"
            n332 = Unbundle By Name(w888) -> ("Self Reference"=w886:refnum<class "LockinDAQ.lvclass">, "AO"=w881:waveform(dbl)[], "SweepResults [i]"=w879:T6, "SweepResults []"=w878:T6)
            n333 = call "AddParametersToSweepResults.vi"("error in (no error)"=w883, "SweepResults [i]"=w879, "AO"=w881, "LockinDAQ in"=w886) -> ("error out"=w884:errorcluster, "SweepResults [i] out"=w880:T6, "LockinDAQ out"=w885:refnum<class "LockinDAQ.lvclass">)  [unwired: 5 in]
            n334 = call "ConcatenateSweepResults.vi"("error in (no error)"=w884, "SweepResults [i]"=w880, "SweepResults []"=w878, "LockinDAQ in"=w885) -> ("error out"=w882:errorcluster, "SweepResults [] out"=w887:T6)  [unwired: 5 in, 1 out]
            n335 = Bundle By Name(cluster=w888, "SweepResults []"=w887) -> (w889:T13)
            n336 = call <vilib>:"Add State(s) to Queue__jki_lib_state_machine.vi"("State(s) in (\"\")"=w892) -> ("States Out"=w891:string)  [unwired: 14 in]
          }
          frame "Sweep: Stop" {
            w894 = State-enum."started" ("state")
            n337 = Unbundle By Name(w905) -> ("Self Reference"=w900:refnum<class "LockinDAQ.lvclass">, "SweepResults []"=w893:T6)
            n338 = call "LockinDAQ.getSweepResults.vi"("error in (no error)"=w898, "getSweepResults"=w893, "LockinDAQ"=w900) -> ("error out"=w897:errorcluster, "LockinDAQ out"=w899:refnum<class "LockinDAQ.lvclass">)  [unwired: 7 in]
            n339 = Unbundle By Name(w899) -> ("Saved Channels: AO"=w901:T18)
            n340 = call "Write Channels_ AO.vi"("error in (no error)"=w897, "Channels: AO"=w901, "LockinDAQ"=w899) -> ("error out"=w903:errorcluster, "LockinDAQ out"=w896:refnum<class "LockinDAQ.lvclass">)  [unwired: 7 in]
            n341 = call "LockinDAQ.getDAQState.vi"("error in (no error)"=w903, "state"=w894, "LockinDAQ"=w896) -> ("error out"=w904:errorcluster, "LockinDAQ out"=w895:refnum<class "LockinDAQ.lvclass">)  [unwired: 7 in]
            n342 = Bundle By Name(cluster=w905, "Self Reference"=w895, "state"=w894, "sweep index"=-1) -> (w906:T13)
            n343 = call <vilib>:"Add State(s) to Queue__jki_lib_state_machine.vi"("State(s) in (\"\")"=w909) -> ("States Out"=w908:string)  [unwired: 14 in]
          }
          frame "---------- Generate ----------" {
            n344 = call <vilib>:"Add State(s) to Queue__jki_lib_state_machine.vi"("State(s) in (\"\")"=w914) -> ("States Out"=w913:string)  [unwired: 14 in]
          }
          frame "Generate: Generate" {
            n345 = local read "measure offset"() -> (w915:bool)
            n346 = Unbundle By Name(w934) -> ("Self Reference"=w923:refnum<class "LockinDAQ.lvclass">)
            n347 = call <userlib>:"Tick Count (ms)__ogtk.vi"("error in (no error)"=w925) -> ("error out"=w921:errorcluster, "millisecond timer value"=w918:u32)  [unwired: 9 in]
            n348 = call "lockin - zero amplitude.vi"("measure\noffset?"=w915, "error in (no error)"=w921, "LockinDAQ"=w923) -> ("error out"=w924:errorcluster, "LockinDAQ out"=w922:refnum<class "LockinDAQ.lvclass">)  [unwired: 7 in]
            n349 = call "LockinDAQ.Generate.Waveforms.vi"("Reset?"="Reset?", "error in (no error)"=w924, "LockinDAQ"=w922) -> ("error out"=w928:errorcluster, "REF []"=w932:waveform(dbl)[], "AO []"=w931:waveform(dbl)[], "LockinDAQ out"=w930:refnum<class "LockinDAQ.lvclass">)  [unwired: 5 in]
            n350 = call "LockinDAQ.getAO.vi"("error in (no error)"=w928, "get AO"=w931, "LockinDAQ"=w930) -> ("error out"=w927:errorcluster, "LockinDAQ out"=w935:refnum<class "LockinDAQ.lvclass">)  [unwired: 7 in]
            n351 = call "LockinDAQ.getREF.vi"("error in (no error)"=w927, "getREF"=w932, "LockinDAQ"=w935) -> ("error out"=w926:errorcluster, "LockinDAQ out"=w929:refnum<class "LockinDAQ.lvclass">)  [unwired: 7 in]
            n352 = call <userlib>:"Tick Count (ms)__ogtk.vi"("error in (no error)"=w926) -> ("error out"=w920:errorcluster, "millisecond timer value"=w919:u32)  [unwired: 9 in]
            n353 = Bundle By Name(cluster=w934, "Self Reference"=w929, "AO"=w931, "REF"=w932) -> (w933:T13)
            n354 = Subtract(x=w919, y=w918) -> (x-y=→"WFM Generation (ms)":u32)
            n355 = call <vilib>:"Add State(s) to Queue__jki_lib_state_machine.vi"("State(s) in (\"\")"=w938) -> ("States Out"=w937:string)  [unwired: 14 in]
          }
        }
      }
    }
    frame Error {
    }
  }
  n356 = call-parent "Process.vi"("error in"=w7, "LevyLab"=w6) -> ("error out"=w4:errorcluster, "LevyLab out"=→"LockinDAQ out":refnum<class "LockinDAQ.lvclass">)  [unwired: 8 in]
  n357 = Merge Errors(w4, w3) -> (→"error out":errorcluster)
